vi "Create_Trajectory_Using_TrajectoryLibrary.vi"() -> ()   [LabVIEW 2019]
doc: "This utility creates trajectories based on the robot configuration, constraints and defined waypoints."
uses:
  <vilib>/Rock Robotics/WPI/ThirdParty/JAS_Junk/TrajLib/Trajectory_Library.lvlib
  <vilib>/Utility/xml.llb/Write to XML File(string).vi
  <vilib>/Rock Robotics/WPI/ThirdParty/JAS_Junk/TrajLib/TRANSLATION2D.ctl
  <vilib>/Rock Robotics/WPI/ThirdParty/JAS_Junk/TrajLib/ROTATION2D.ctl
  <vilib>/Rock Robotics/WPI/ThirdParty/JAS_Junk/TrajLib/POSE2D.ctl
  <vilib>/Rock Robotics/WPI/ThirdParty/JAS_Junk/TrajLib/TRAJ_STATE.ctl
  <vilib>/Rock Robotics/WPI/ThirdParty/JAS_Junk/TrajLib/TRAJECTORY.ctl
  <vilib>/Utility/xml.llb/Read From XML File(string).vi
  <vilib>/Rock Robotics/WPI/ThirdParty/JAS_Junk/TrajLib/UTIL_WEIGHTED_WAYPOINT.ctl
  <vilib>/Rock Robotics/WPI/ThirdParty/JAS_Junk/TrajLib/DIFF_DRIVE_KINEMATICS.ctl
  <vilib>/Rock Robotics/WPI/ThirdParty/JAS_Junk/TrajLib/TRAJ_CONSTRAINT_DIIF_DRIVE_KINEMATICS.ctl
  <vilib>/Rock Robotics/WPI/ThirdParty/JAS_Junk/TrajLib/TRAJ_CONSTRAINT_CENTRIPETAL_ACCEL.ctl
  <vilib>/Analysis/Matrix/Datatypes/RealMatrix.ctl
  <vilib>/Analysis/Matrix/NI_Matrix.lvlib
  <vilib>/Rock Robotics/WPI/ThirdParty/JAS_Junk/TrajLib/SWERVE_DRIVE_KINEMATICS.ctl
  <vilib>/Rock Robotics/WPI/ThirdParty/JAS_Junk/TrajLib/TRAJ_CONSTRAINT_SWERVE_DRIVE_KINEMATICS.ctl
  <vilib>/Rock Robotics/WPI/ThirdParty/JAS_Junk/TrajLib/SIMPLE_MOTOR_FF.ctl
  <vilib>/Rock Robotics/WPI/ThirdParty/JAS_Junk/TrajLib/TRAJ_CONSTRAINT_DIIF_DRIVE_VOLTAGE.ctl
  <vilib>/Rock Robotics/WPI/ThirdParty/JAS_Junk/TrajLib/MECA_DRIVE_KINEMATICS.ctl
  <vilib>/Rock Robotics/WPI/ThirdParty/JAS_Junk/TrajLib/TRAJ_CONSTRAINT_MECA_DRIVE_KINEMATICS.ctl
  <vilib>/Rock Robotics/WPI/ThirdParty/JAS_Junk/TrajLib/TRAJ_CONFIG.ctl
  TrajCreateUnitsENUM.ctl
  TrajCreateConfig.ctl
panel:
  in  "End Program":bool
  in  "Tab Control":T1(tab)
  out "Config File Read\nWithout Error":bool
  out "Config File  Read Error":errorcluster
  out "Read Config File Comment":string
  in  "Read Config File Name":path
  in  "ReadConfigFile":bool
  in  "Field Selector":string(combo)
  in  "Units Selector":T2
  in  "MaxVelocity":dbl=50.0 format="%17.1f"
  in  "MaxAcceleration":dbl=40.0 format="%17.1f"
  out "MaxVelocity M/S":dbl=2.0 format="%17.4f"
  out "MaxAcceleration M/S^2":dbl=1.3 format="%17.4f"
  in  "Right Rear":T3={"X"=-0.5, "Y"=0.5} {"Y" format="%14.3f"; "X" format="%14.3f"}
  in  "Left Rear":T3={"X"=-0.5, "Y"=-0.5} {"Y" format="%14.3f"; "X" format="%14.3f"}
  in  "Right Front":T3={"X"=0.5, "Y"=0.5} {"Y" format="%14.3f"; "X" format="%14.3f"}
  in  "Left Front":T3={"X"=0.5, "Y"=-0.5} {"Y" format="%14.3f"; "X" format="%14.3f"}
  in  "Use Centripetal\nAcceleration\nConstaint":bool=TRUE
  out "Max Cent Accel M/S^2":dbl=1.0 format="%20.4f"
  in  "Max Cent Accel":dbl=20.0 format="%20.1f"
  in  "Use Diff Drive\nKinematic\nConstraint":bool=TRUE
  out "Wheelbase Width M":dbl=0.66 format="%20.4f"
  in  "Wheelbase Width":dbl=20.866 format="%20.1f"
  in  "Max Voltage":dbl=12.0 format="%20.4f"
  in  "SIMPLE_MOTOR_FF":T4={"Ks"=0.9, "Kv"=8.74, "Ka"=1.92} {"Ka" format="%13.4f"; "Kv" format="%13.4f"; "Ks" format="%13.4f"}
  in  "Use Diff Drive\nVoltage\nConstraint":bool=TRUE
  in  "Wheels":T3[](array[typedef])=[{"X"=0.5, "Y"=-0.5}, {"X"=0.5, "Y"=0.5}, {"X"=-0.5, "Y"=0.5}, {"X"=-0.5, "Y"=-0.5}] {"Y" format="%14.3f"; "X" format="%14.3f"}
  in  "Use Swerve Drive\nKinematics\nConstraint":bool
  in  "Use Mecanum \nDrive Kinematics\nConstraint":bool
  out "Left Front M":T3 {"Y" format="%14.3f"; "X" format="%14.3f"}
  out "Right Front M":T3 {"Y" format="%14.3f"; "X" format="%14.3f"}
  out "Left Rear M":T3 {"Y" format="%14.3f"; "X" format="%14.3f"}
  out "Right Rear M":T3 {"Y" format="%14.3f"; "X" format="%14.3f"}
  out "SIMPLE_MOTOR_FF M":T4 {"Ka" format="%13.4f"; "Kv" format="%13.4f"; "Ks" format="%13.4f"}
  out "Wheels M":T3[](array[typedef]) {"Y" format="%14.3f"; "X" format="%14.3f"}
  in  "WayPoints":T5[](array[typedef])=[{"X"=15.0, "Y"=105.0, "ANGLE"=-45.0, "WEIGHT"=12.0}, {"X"=105.0, "Y"=65.0, "ANGLE"=0.0, "WEIGHT"=12.0}, {"X"=210.0, "Y"=106.0, "ANGLE"=45.0, "WEIGHT"=12.0}, {"X"=350.0, "Y"=105.0, "ANGLE"=-45.0, "WEIGHT"=12.0}] {"WEIGHT" format="%13.3f"; "ANGLE" format="%13.3f"; "Y" format="%13.3f"; "X" format="%13.3f"}
  in  "Spline Type":enum32{"Radio Selection 1", "Radio Selection 2"}(radio)
  in  "Reverse":bool
  in  "UseWeights":bool
  in  "Calculate\nTrajectory":bool
  out "Trajectory\nCompleted\nError Free":bool
  out "Trajectory calculation error":errorcluster
  out "Position":cluster{dbl[], dbl[]}[](graph)
  out "Field Display":T6(plugin-control)
  out "Trajectory Data":cluster{dbl[], dbl[]}[](graph)
  out "differential \ndrive \nmax speed":dbl format="%15.1f"
  out "Traj States\nSize":i32
  out "Trajectory States":T7[](array[typedef]) {"POSE"."ROTATION"."SIN" format="%13.4f"; "POSE"."ROTATION"."COS" format="%13.4f"; "POSE"."ROTATION"."VALUE" format="%13.4f"; "POSE"."TRANSLATION"."Y" format="%14.3f"; "POSE"."TRANSLATION"."X" format="%14.3f"}
  in  "Trajectory JSON File Name":path
  out "JSON File Saved\nWithout Error":bool
  out "Write CSV File Error":errorcluster
  in  "PathWeaver Length Units":T10(radio)
  in  "WriteJSONFile":bool
  out "CSV File Saved\nWithout Error":bool
  in  "Trajectory Type":enum32{"Radio Selection 1", "Radio Selection 2"}(radio)
  out "Write Trajectory\nFile Error":errorcluster
  in  "Trajectory File Comment":string
  in  "Trajectory CSV File Name":path
  in  "WriteTrajFile":bool
  out "Config File Saved\nWithout Error":bool
  out "Write Config FIle Error":errorcluster
  in  "Write Config File Comment":string
  in  "Write Config File Name":path
  in  "WriteConfigFile":bool
  # "Create Trajectory  (Use LabVIEW trajectory library)"
  # "Instructions:  \n----------------\n\nThis utility will create a trajectory, show the data on the various tabs, and optionally write a \"field absolute\" or \"robot relative\" trajectory to a file. \nTo use this utility:\n\n1) Read all of these instructions!\n2) Define the robot's physical data on the \"Robot Data\" tab.  \n3) Define the robot's movement constraints on the \"Constraints\" page.  \n4) Define the trajectory on the \"Define/Create Trajectory\" tab.  These are the beginning and ending positions/headings, and internal positions/headings.  \n    Cubic splines only use the first and last \"angle\".  The other internal \"angles\" are calculated.  Quintic splines use all the defined angles.\n5) Press the \"Calculate Trajectory\".  If a good trajectory was calculated it will be displayed.  If no errors are generated the Trajectory Complete\n    light will be on.  Errors will be displayed in the error indicator.  The path can be recalculated many times before performing any other action.\n\nAfter a Trajectory has been calculated, the \"trajectory can be written to a file.  The absolute path is converted to a robot relative trajectory.  To do this:\n1) Enter a comment to be included in the file.  Anything can be entered.\n2) Select the file name.\n3) Press \"Create Trajectory File\"  If an error occurs it will be displayed in the File Creation Error indicator.\n\nNotes:\n--------\n- All the robot parameters, path, and field dimensions are in UNITS, and DEGREES.  Select UNITS from the \"Robot Data\" page.  The resulting  \n  trajectory is converted to METERS, and RADIANS to match the rest of this library!\n- The trajectory library is the same as the WPILIB spline and trajectory library for Java and C++.\n- 2019 playing field size - width: 26 ft 11.25 In = 323.25 in , length: 52 ft 5.25 in = 629.25 in  (I didn't verify this for the 2020 version.)"
  # "Read Trajectory Waypoints and Configuration from File"
  # "ROBOT DATA"
  # "UNITS/SEC"
  # "Meters/SEC"
  # "UNITS/SEC^2"
  # "Meters/SEC^2"
  # "Simulated robot max speed is: 68.266 Inches/Second"
  # "UTILITY CONFIGURATION"
  # "Diff Kinematics Constraint"
  # "Centripetal Accel Constraint"
  # "Diff Voltage Constraint"
  # "UNITS"
  # "UNITS/SEC^2"
  # "VOLTS"
  # "METERS"
  # "METERS/SEC^2"
  # "Distance is:\nUNITS"
  # "Simulated robot wheelbase is 20.87 in"
  # "Ks = Volts\nKv = VoltSec/Meter\nKa = Volt(Sec^2)/Meter"
  # "Swerve Kinematics Constraint"
  # "Mechanum Kinematics Constraint"
  # "Values\nare \nUNITS"
  # "Values\nare \nUNITS"
  # "TRAJECTORY DEFINITION"
  # "To delete array elements or the entire array, right click on the array or element, select Data Operations, then select the action to be performed."
  # "UNITS, UNITS, DEGREES, SCALAR"
  # "INCHES/SEC"
  # "Write Trajectory to File   -   CSV, and / or JSON"
  # "Write Trajectory Waypoints and Configuration to File"
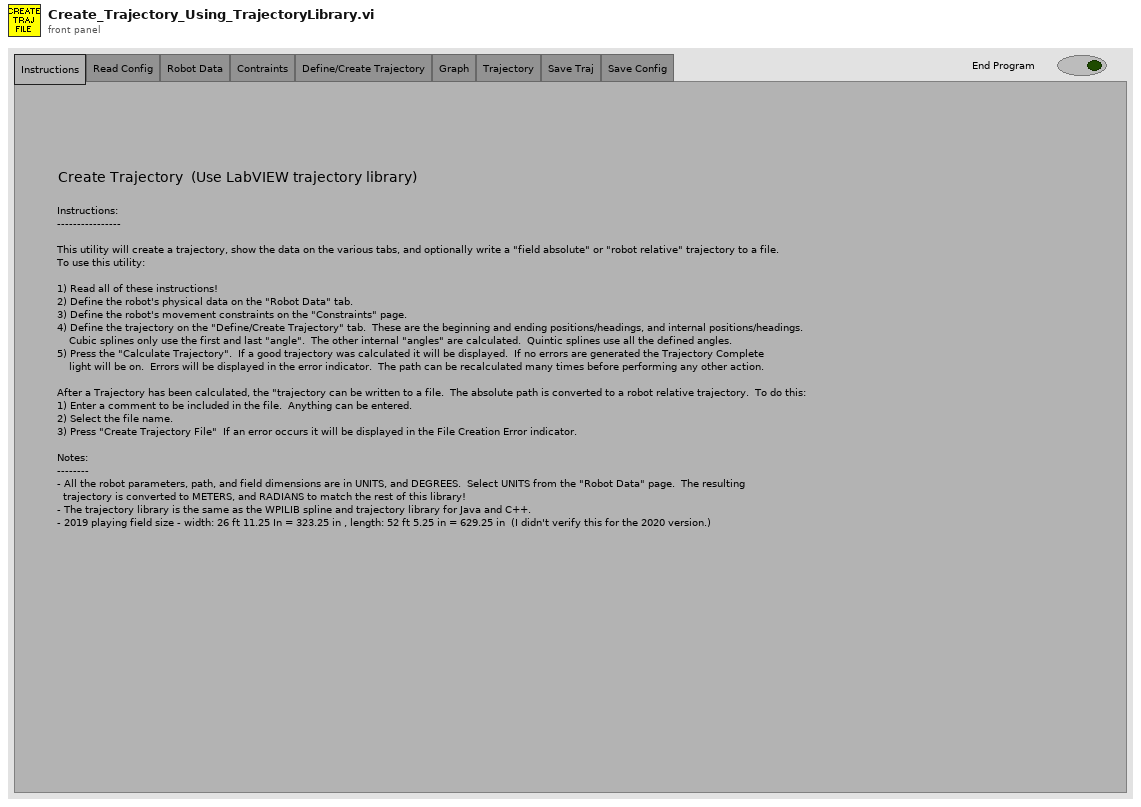
[diagram p1: front panel]
types:
  T1 = enum32{"Instructions", "Read Config", "Robot Data", "Contraints", "Define/Create Trajectory", "Graph", "Trajectory", "Save Traj", "Save Config"}
  T2 = typedef "TrajCreateUnitsENUM.ctl" = enum16{"Inches", "Feet", "Centimeters", "Meters"}
  T3 = typedef "Trajectory_Library.lvlib/TRANSLATION2D.ctl" = cluster{"X":dbl, "Y":dbl}
  T4 = typedef "Trajectory_Library.lvlib/SIMPLE_MOTOR_FF.ctl" = cluster{"Ks":dbl, "Kv":dbl, "Ka":dbl}
  T5 = typedef "Trajectory_Library.lvlib/UTIL_WEIGHTED_WAYPOINT.ctl" = cluster{"X":dbl, "Y":dbl, "ANGLE":dbl, "WEIGHT":dbl}
  T6 = typedef "IMAQ Image.ctl" = refnum<image>
  T7 = typedef "Trajectory_Library.lvlib/TRAJ_STATE.ctl" = cluster{"TimeSeconds":dbl, "Velocity":dbl, "Acceleration":dbl, "POSE":T8, "Curvature":dbl}
  T8 = typedef "Trajectory_Library.lvlib/POSE2D.ctl" = cluster{"TRANSLATION":T3, "ROTATION":T9}
  T9 = typedef "Trajectory_Library.lvlib/ROTATION2D.ctl" = cluster{"VALUE":dbl, "COS":dbl, "SIN":dbl}
  T10 = enum32{"Radio Selection 1", "Radio Selection 2", "Radio Selection 3", "Radio Selection 4", "Radio Selection 5"}
  T11 = typedef "Image Type" = u32
  T12 = enum8{"Enabled", "Disabled", "Disabled and Grayed Out"}
  T13 = typedef "Trajectory_Library.lvlib/TRAJECTORY.ctl" = cluster{"TotalTImeSecs":dbl, "States":T7[]}
  T14 = typedef "TrajCreateConfig.ctl" = cluster{"Write Config File Name":path, "Write Config File Comment":string, "WayPoints":T5[], "TRAJECTORY_CONFIG":T15, "IsCubic":bool, "Units Selector":T2, "UseWeights":bool}
  T15 = typedef "Trajectory_Library.lvlib/TRAJ_CONFIG.ctl" = cluster{"MaxVelocity":dbl, "Max Acceleration":dbl, "StartVelocity":dbl, "End Velocity":dbl, "Reversed":bool, "DiffDrKineConstntDefined":bool, "CentAcellConstntDefined":bool, "DiffDrVoltConstntDefined":bool, "DIFF_DRIVE_KINE_CONSTRAINT":T16, "CENTRIPETAL_ACCEL_CONSTRAINT":T18, "SwerveDrKineConstntDefined":bool, "SWERVE_DRIVE_KINE_CONSTRAINT":T19, "DIFF_DRIVE_VOLTAGE_CONSTRAINT":T22, "MECANUM_DRIVE_KINE_CONSTRAINT":T23, "MecanumDrKineConstntDefined":bool}
  T16 = typedef "Trajectory_Library.lvlib/TRAJ_CONSTRAINT_DIIF_DRIVE_KINEMATICS.ctl" = cluster{"Max Speed (M/S)":dbl, "DIFF_DRIVE_KINEMATICS":T17}
  T17 = typedef "Trajectory_Library.lvlib/DIFF_DRIVE_KINEMATICS.ctl" = cluster{"TrackWidth_Meters":dbl}
  T18 = typedef "Trajectory_Library.lvlib/TRAJ_CONSTRAINT_CENTRIPETAL_ACCEL.ctl" = cluster{"Max Cent Accel":dbl}
  T19 = typedef "Trajectory_Library.lvlib/TRAJ_CONSTRAINT_SWERVE_DRIVE_KINEMATICS.ctl" = cluster{"Max Speed (M/S)":dbl, "SwerveKinematics":T20}
  T20 = typedef "Trajectory_Library.lvlib/SWERVE_DRIVE_KINEMATICS.ctl" = cluster{"NumModules":i32, "InverseKinematics":T21, "ForwardKinematics":T21, "Modules":T3[], "PrevCoR":T3}
  T21 = typedef "NI_Matrix.lvlib/RealMatrix.ctl" = dbl[][]
  T22 = typedef "Trajectory_Library.lvlib/TRAJ_CONSTRAINT_DIIF_DRIVE_VOLTAGE.ctl" = cluster{"Max Voltage":dbl, "DIFF_DRIVE_KINEMATICS":T17, "SIMPLE_MOTOR_FF":T4}
  T23 = typedef "Trajectory_Library.lvlib/TRAJ_CONSTRAINT_MECA_DRIVE_KINEMATICS.ctl" = cluster{"Max Speed (M/S)":dbl, "MECA_DRIVE_KINEMATICS":T24}
  T24 = typedef "Trajectory_Library.lvlib/MECA_DRIVE_KINEMATICS.ctl" = cluster{"FrontLeft":T3, "FrontRight":T3, "RearLeft":T3, "RearRight":T3, "InverseKinematics":T21, "ForwardKinematics":T21, "PrevCoR":T3}
  T25 = typedef "TrajectoryUtils_Field_Info.ctl" = cluster{"FIeld_File_Name":string, "Top_Left_X":i32, "Top_Left_Y":i32, "Bottom_Right_X":i32, "Bottom_Right_Y":i32, "Field_Size_X":dbl, "Field_Size_Y":dbl, "FIeld_Size_Units":string}
  T26 = typedef "Trajectory_Library.lvlib/WEIGHTED_WAYPOINT.ctl" = cluster{"TRANSLATION":T3, "ROTATION":T9, "SCALAR":dbl}
  T27 = typedef "Trajectory_Library.lvlib/SPLINE_CTRL_VECTOR.ctl" = cluster{"Xs":dbl[], "Ys":dbl[]}
  T28 = typedef "Trajectory_Library.lvlib/CHASSIS_SPEEDS.ctl" = cluster{"vX":dbl, "vY":dbl, "vOmega":dbl}
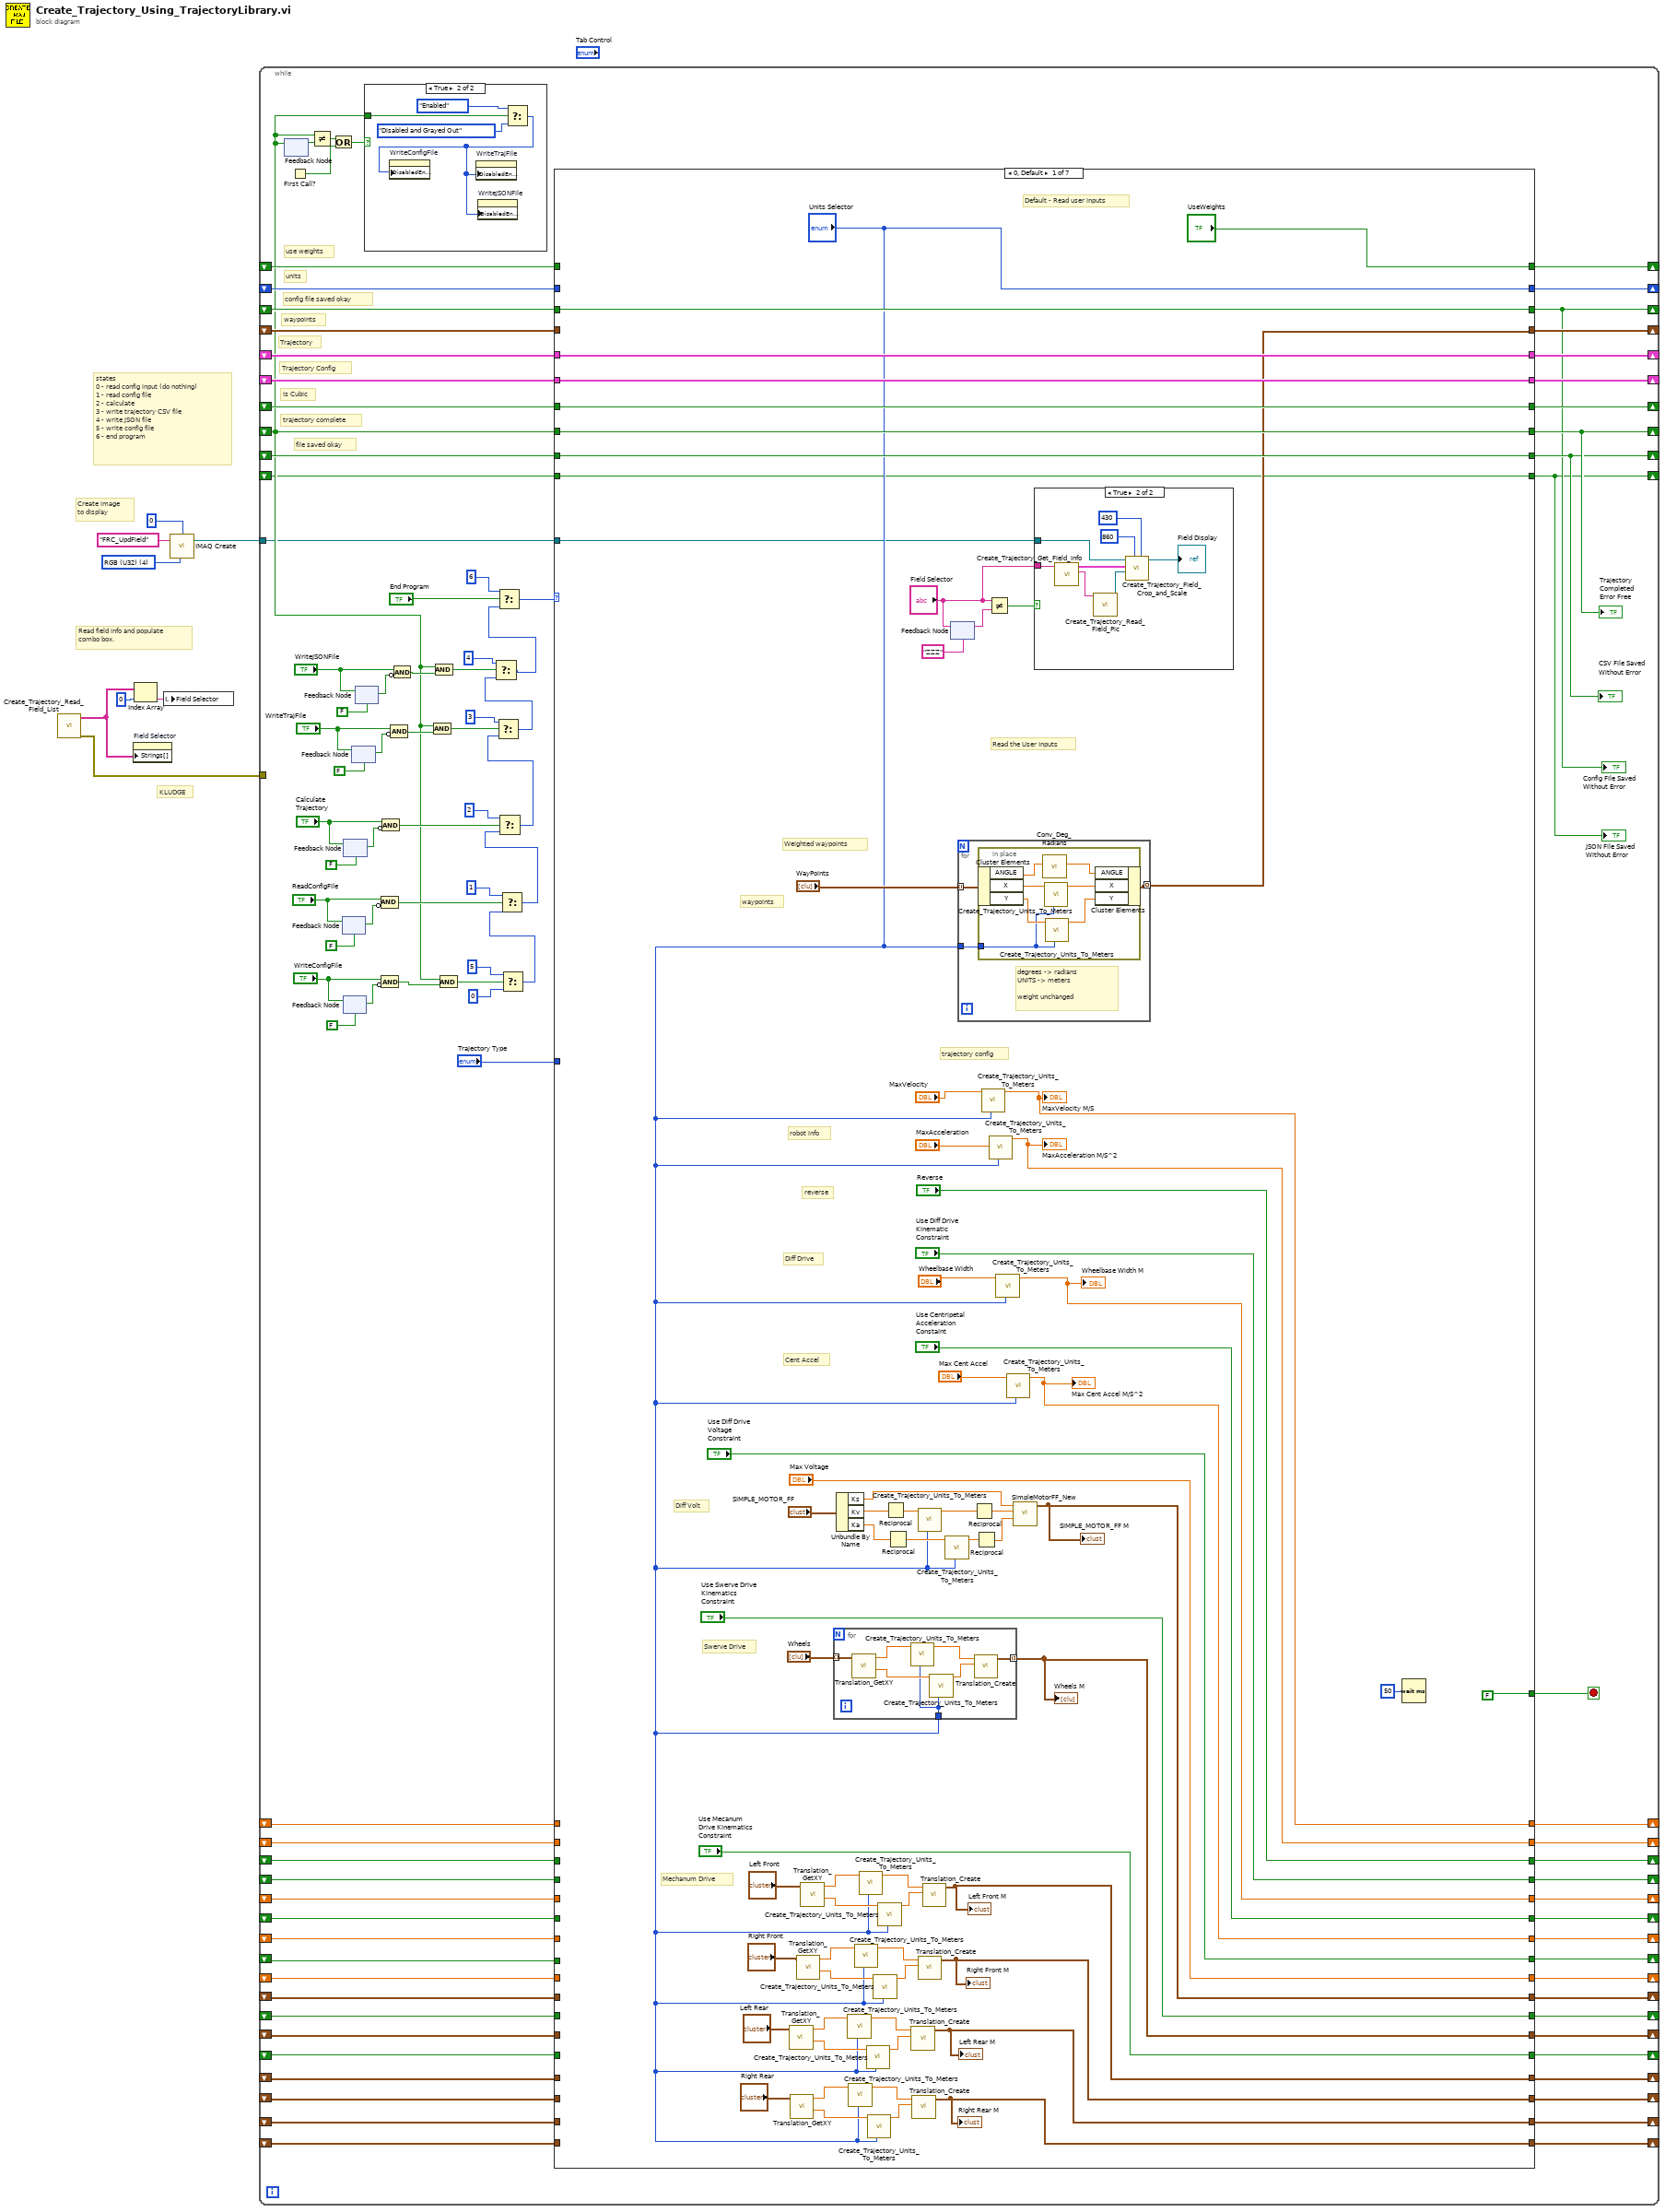
[diagram p0: block diagram]
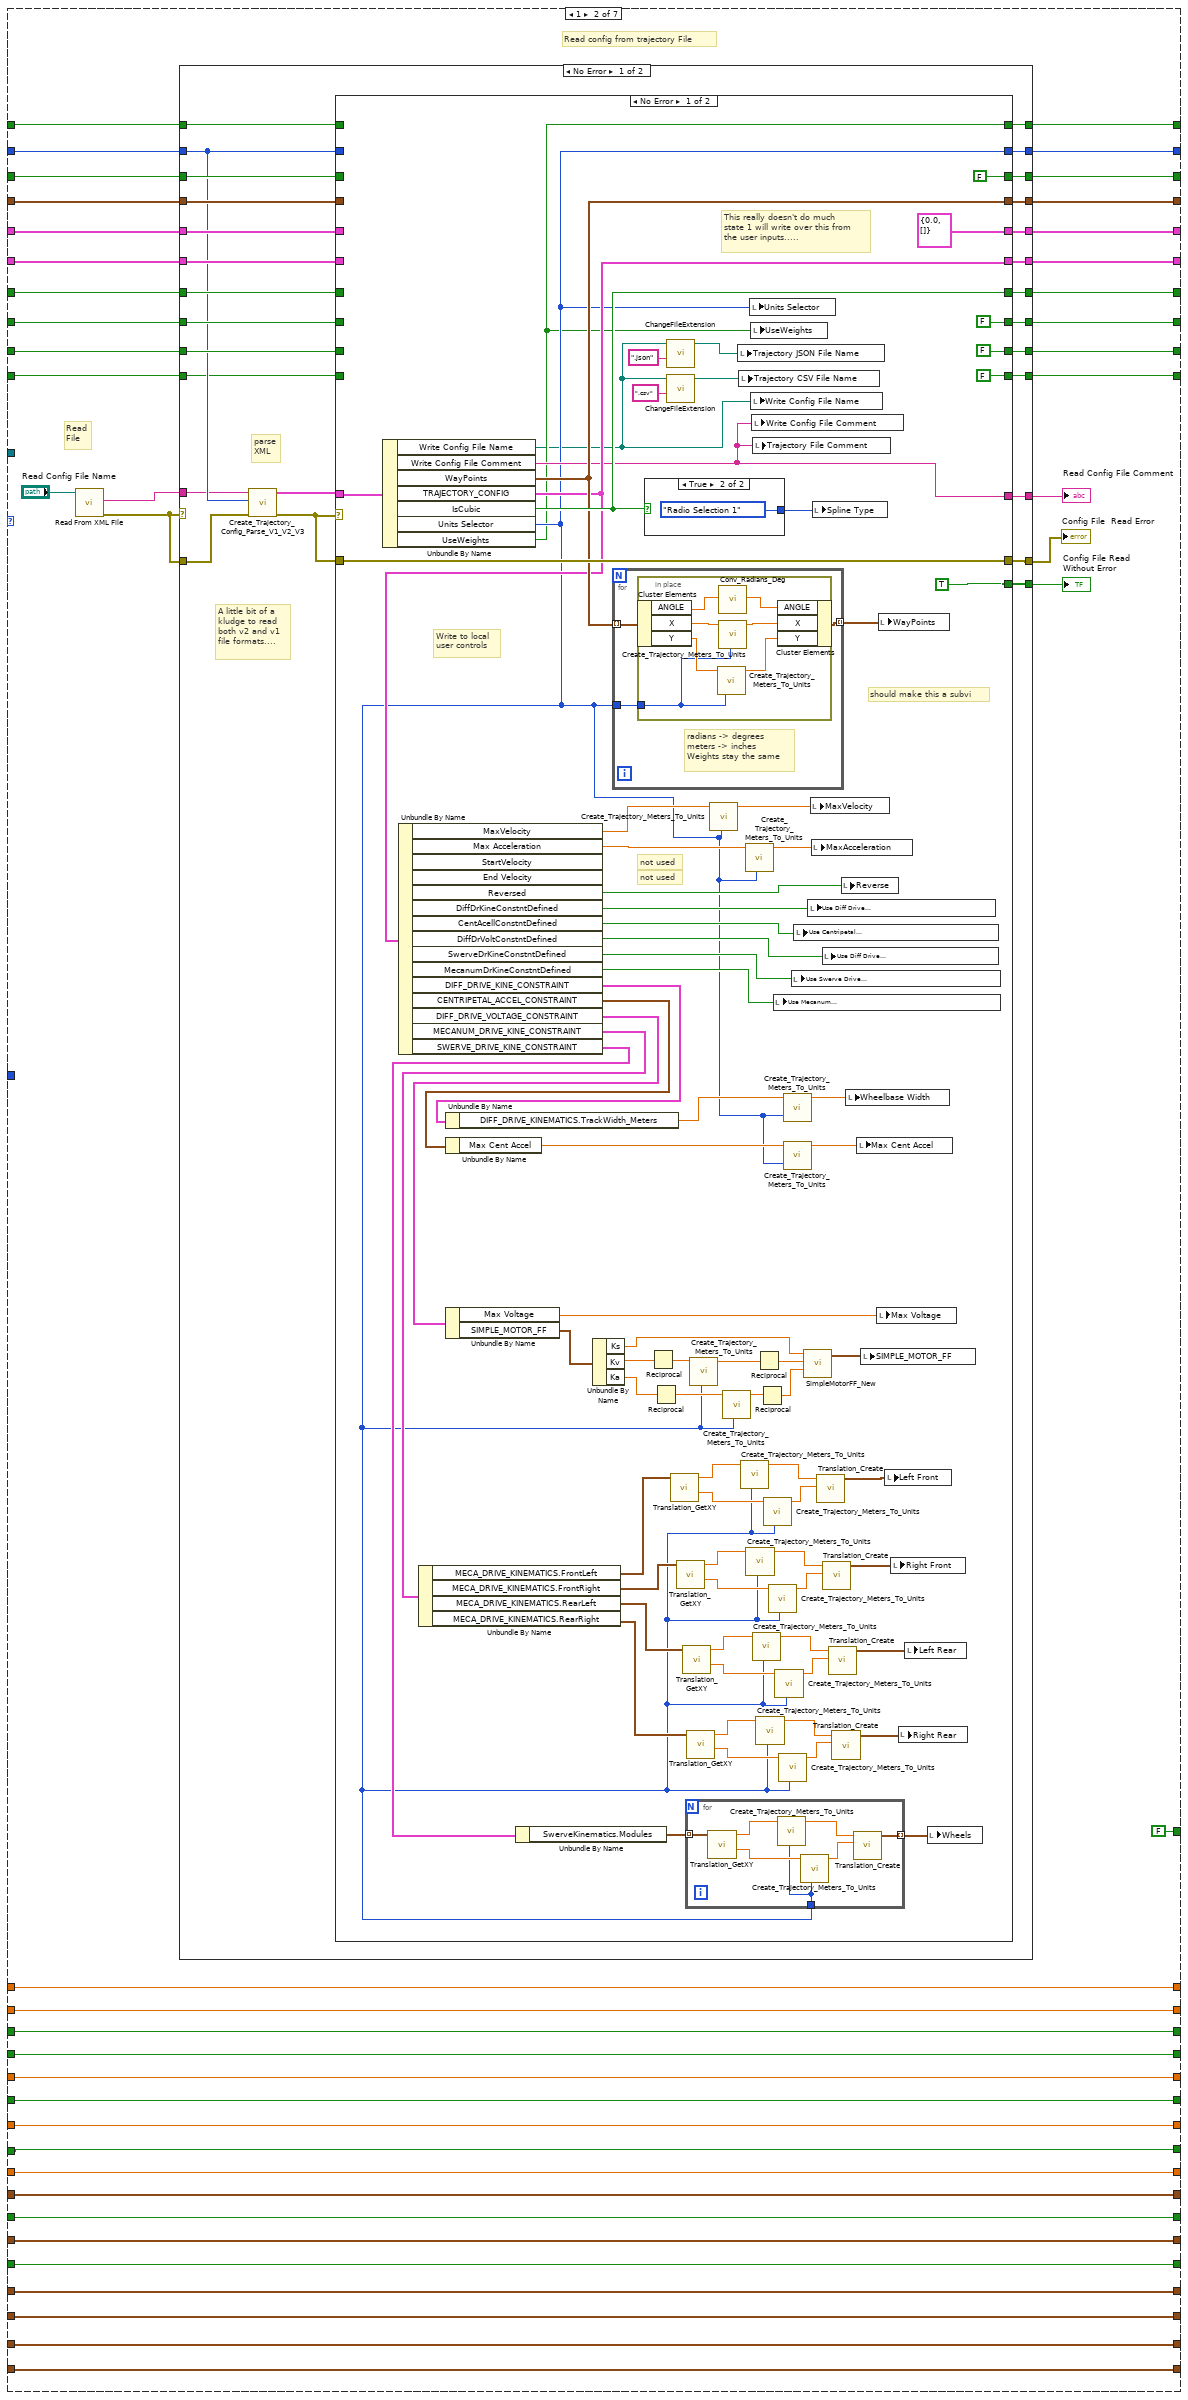
[diagram p4: hidden frame]
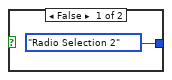
[diagram p5: hidden frame]
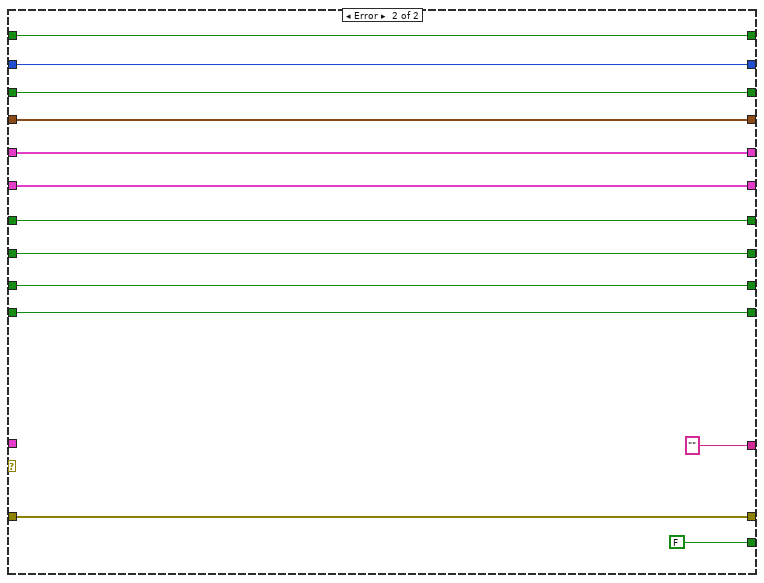
[diagram p6: hidden frame]
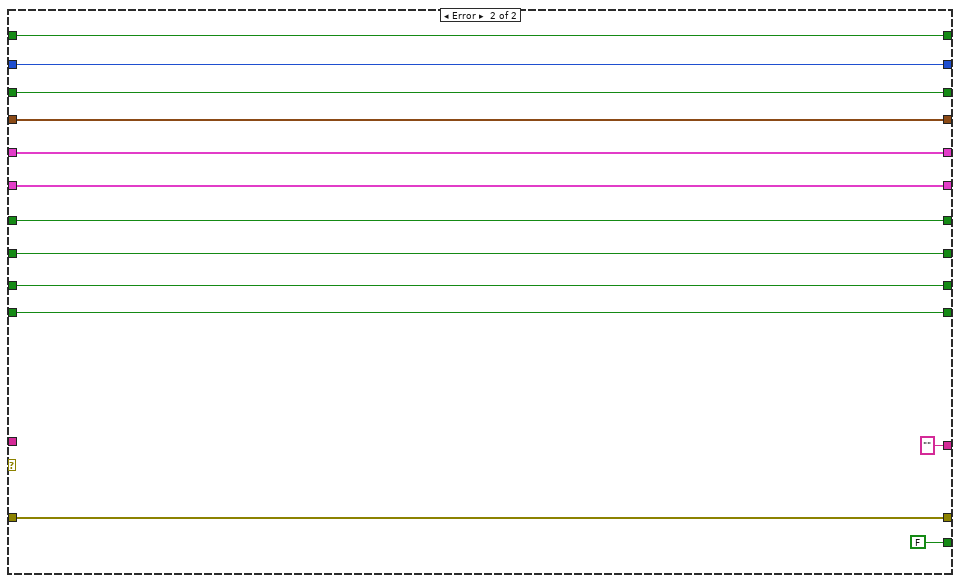
[diagram p7: hidden frame]
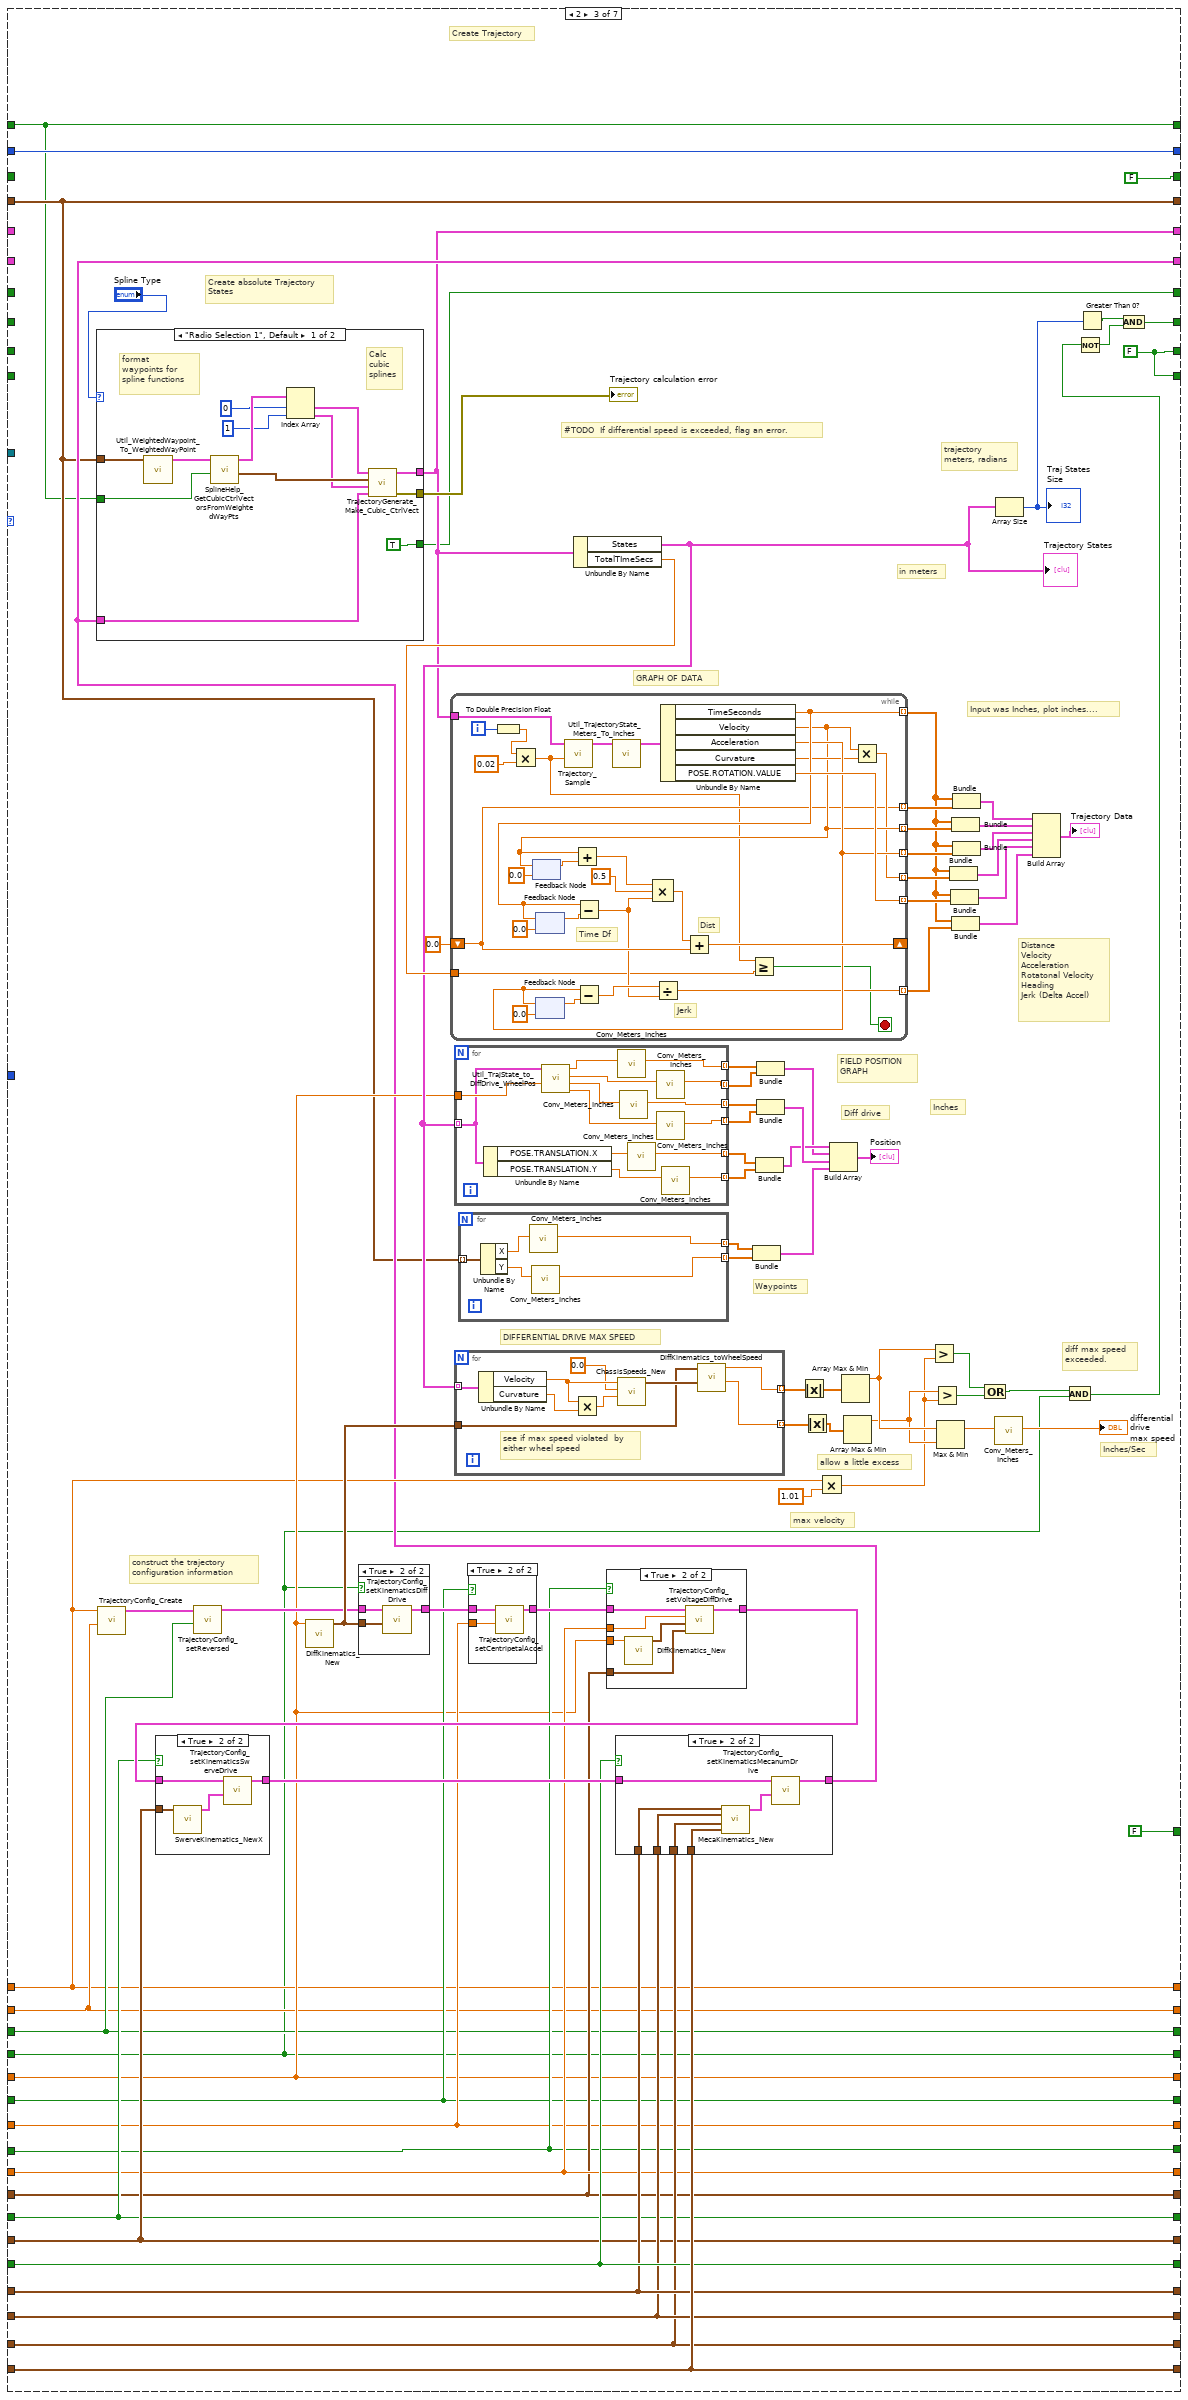
[diagram p8: hidden frame]
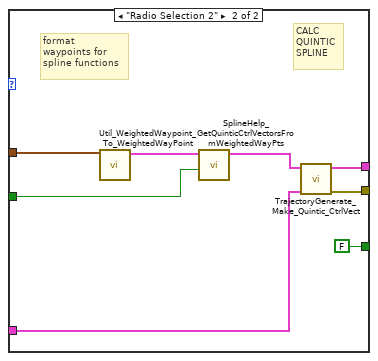
[diagram p12: hidden frame]
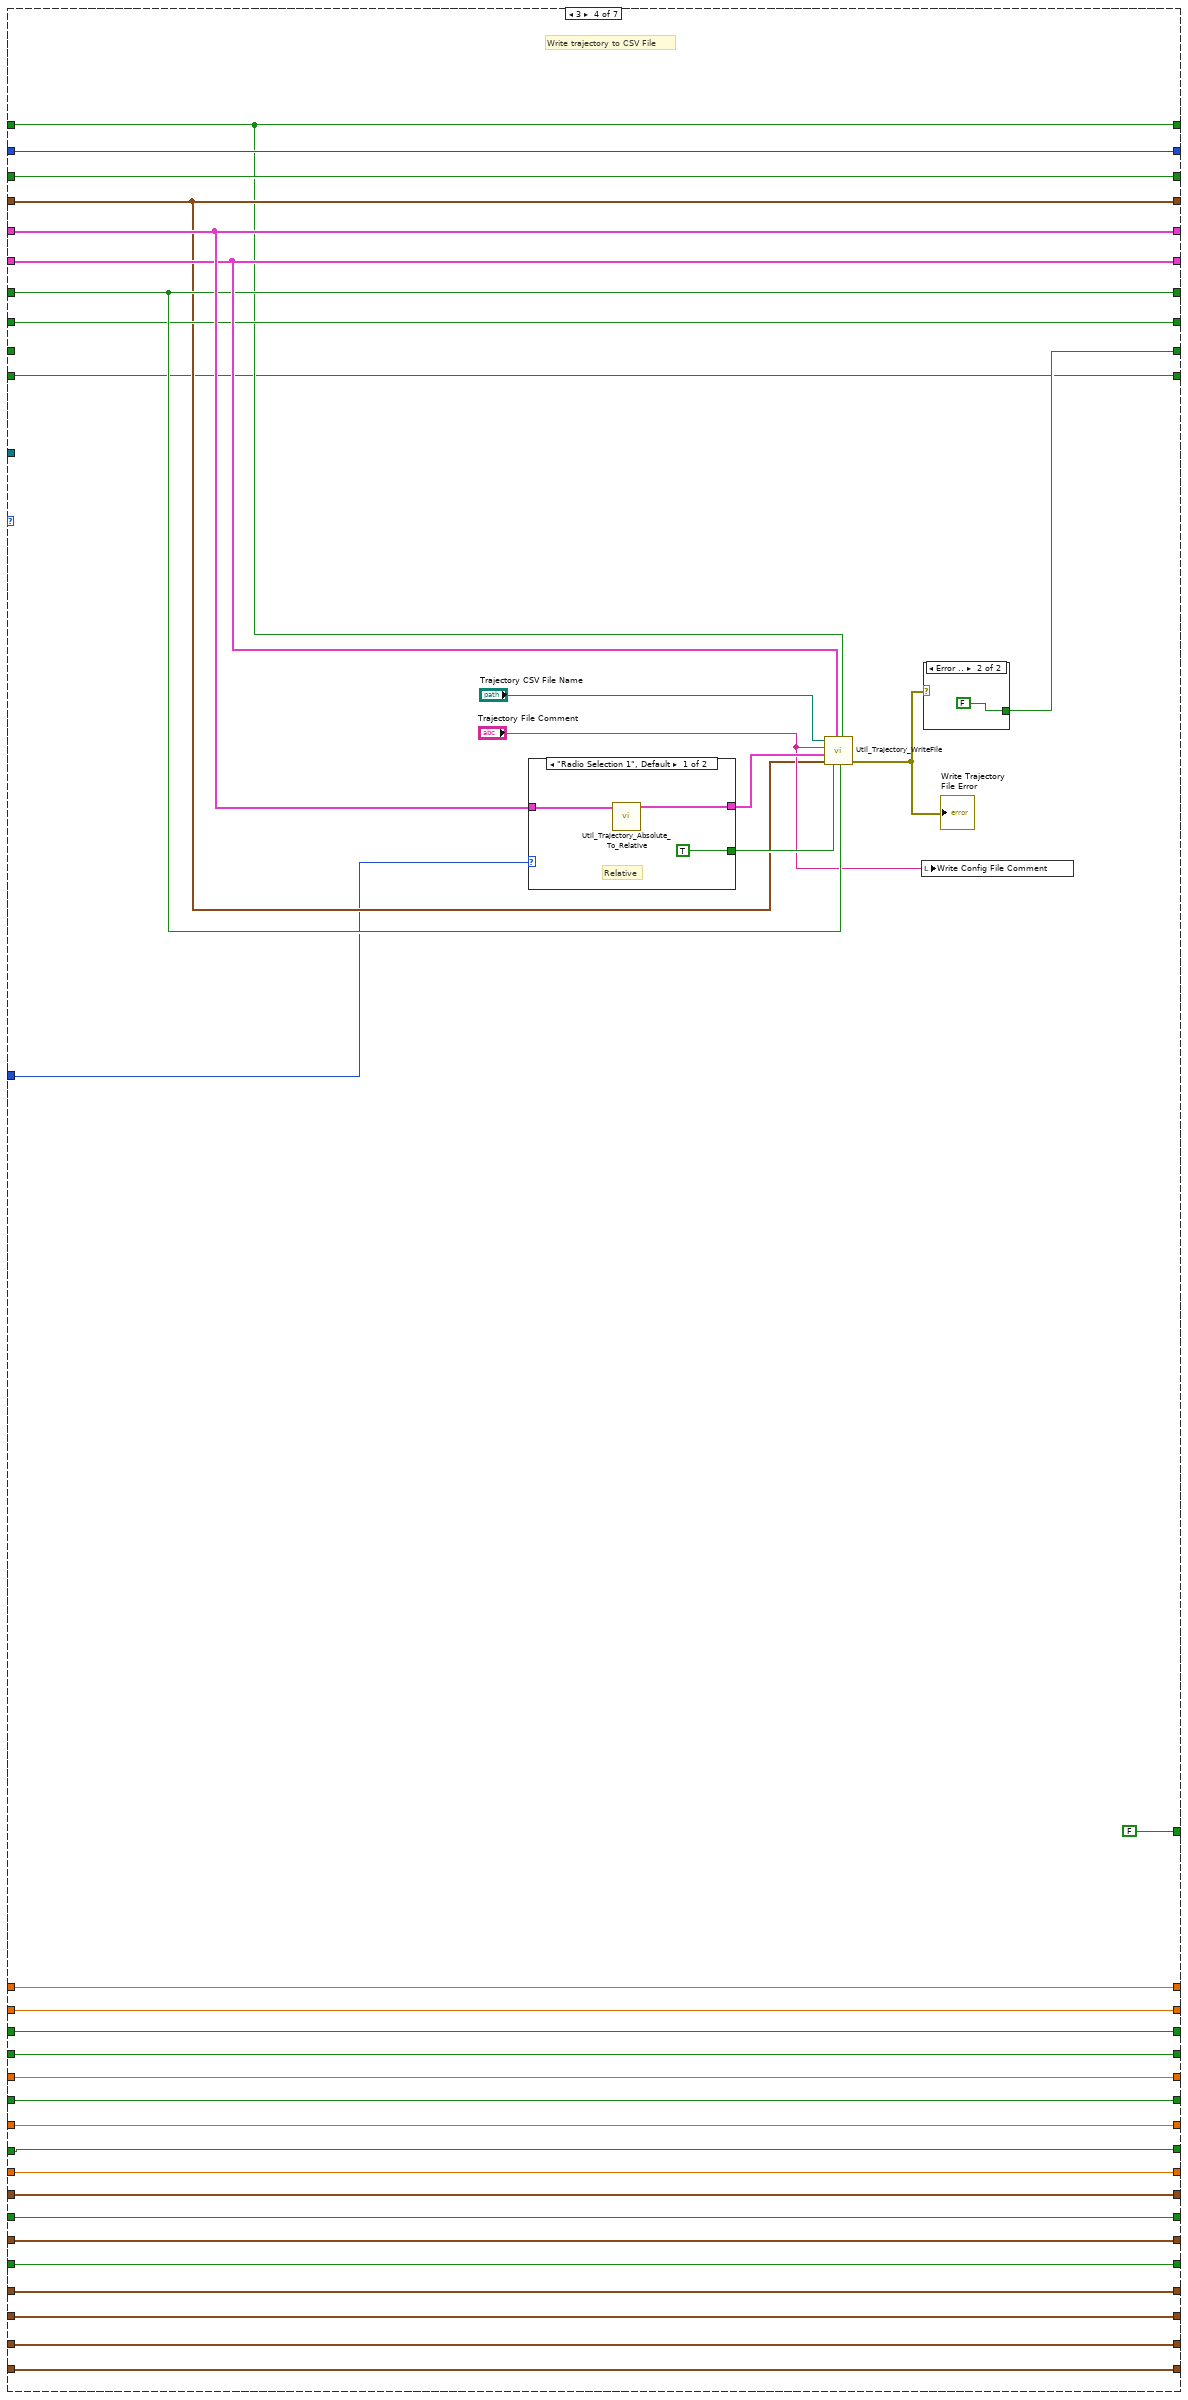
[diagram p15: hidden frame]
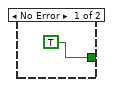
[diagram p16: hidden frame]
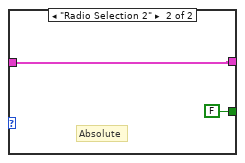
[diagram p17: hidden frame]
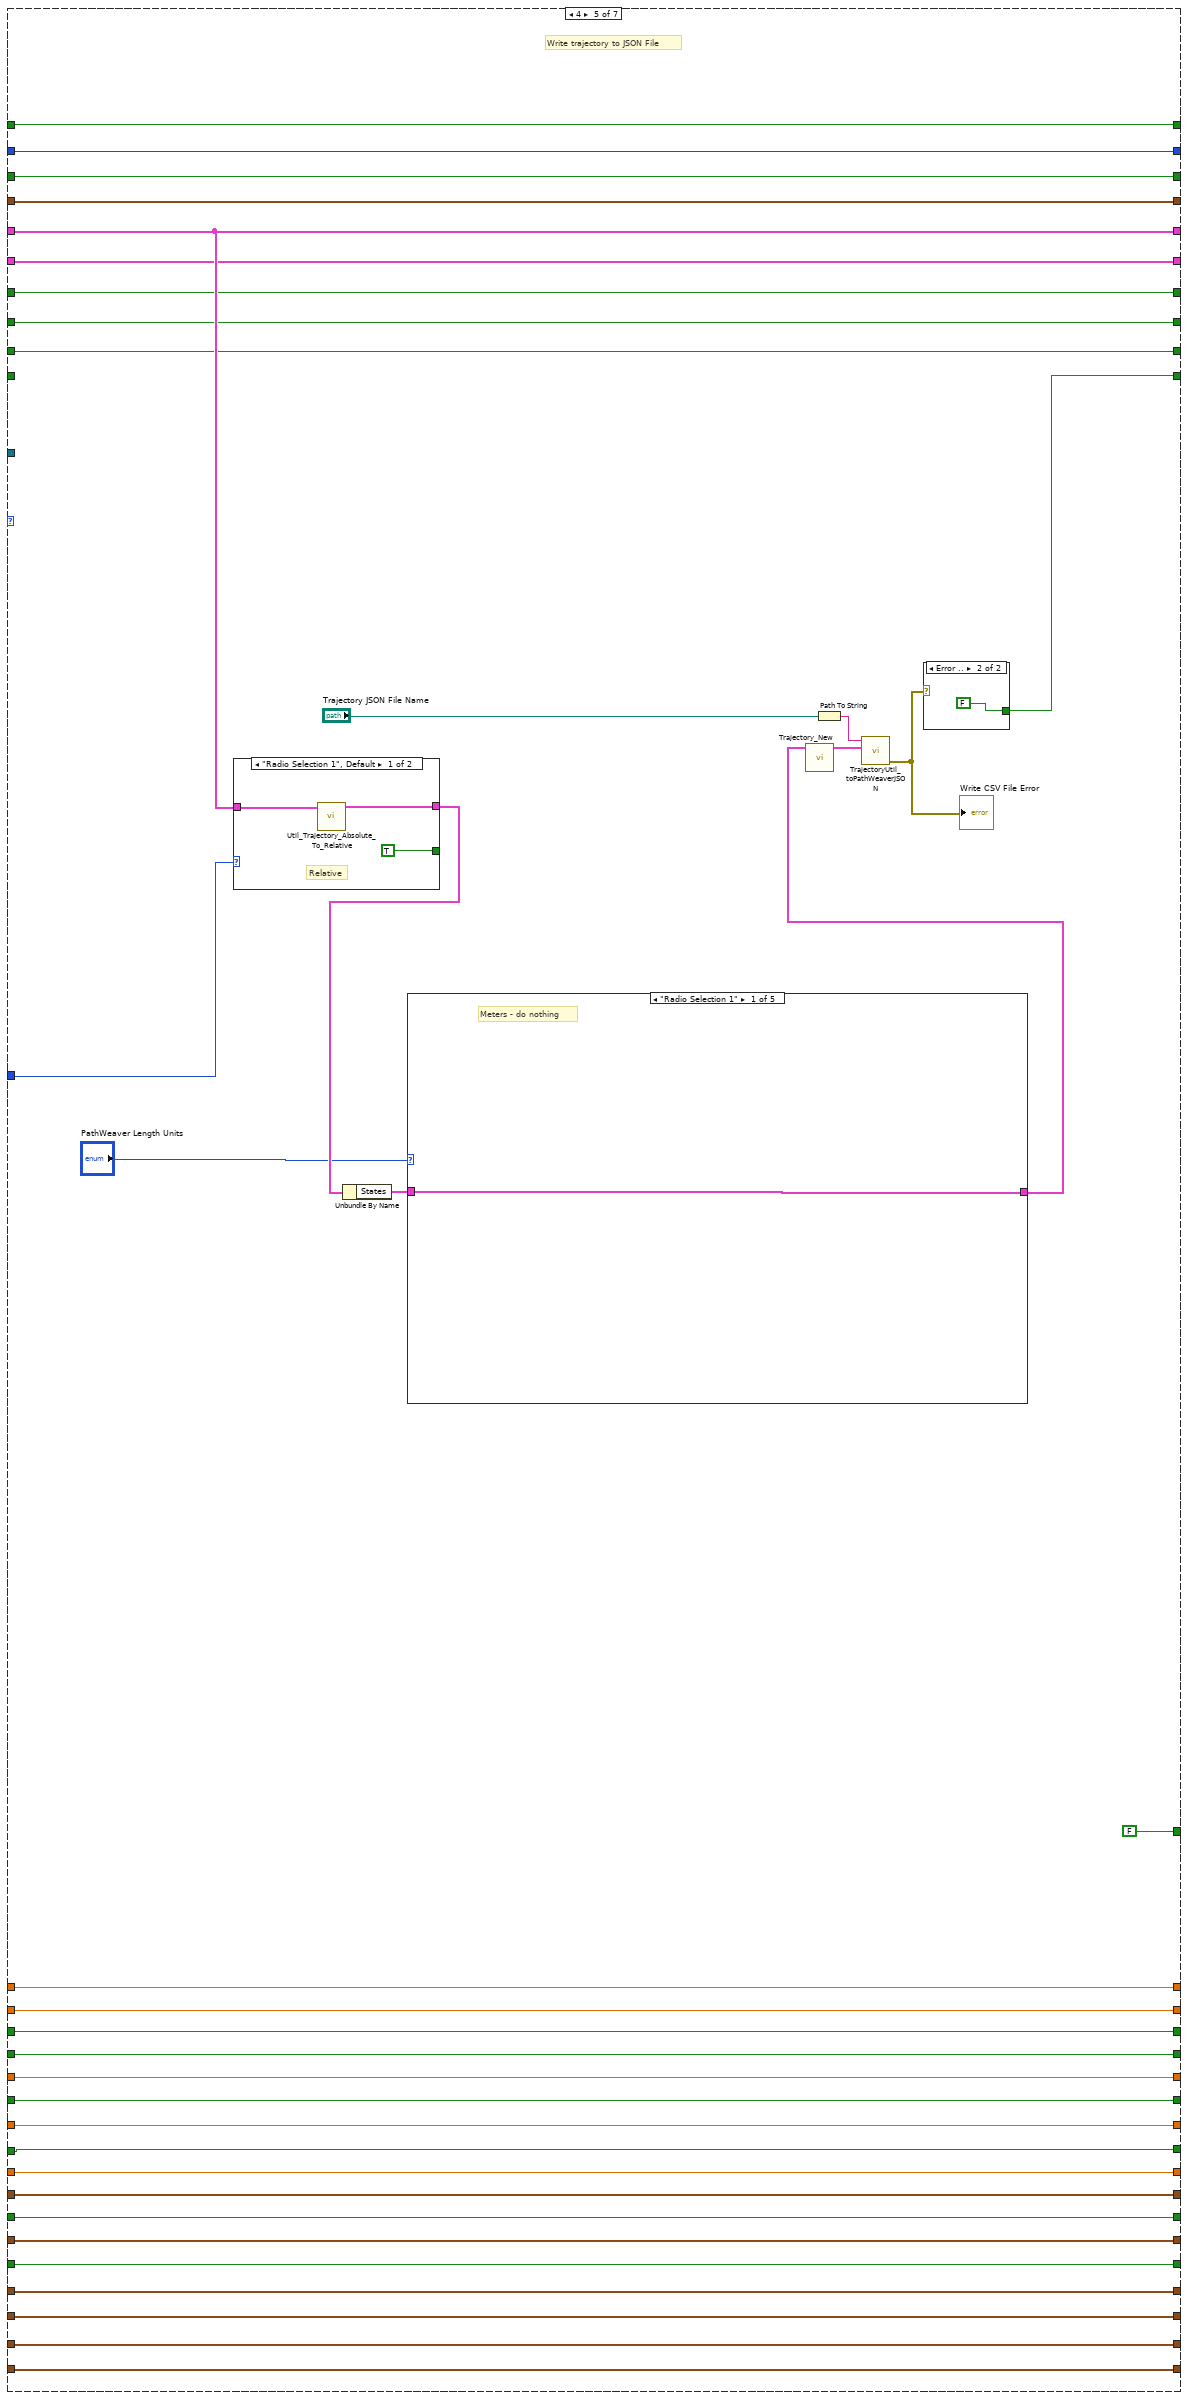
[diagram p18: hidden frame]
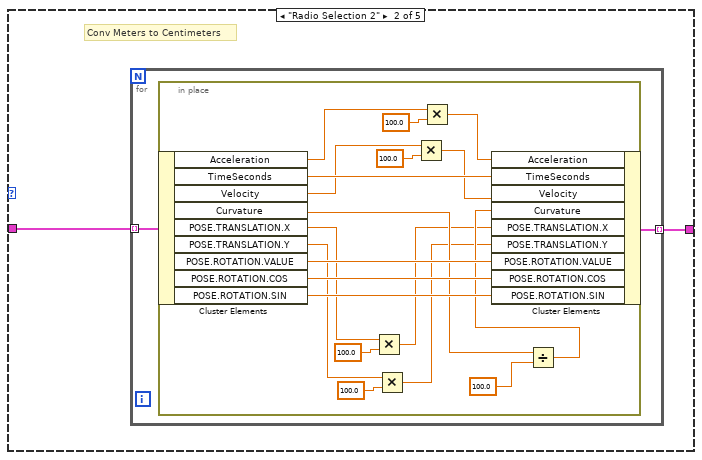
[diagram p19: hidden frame]
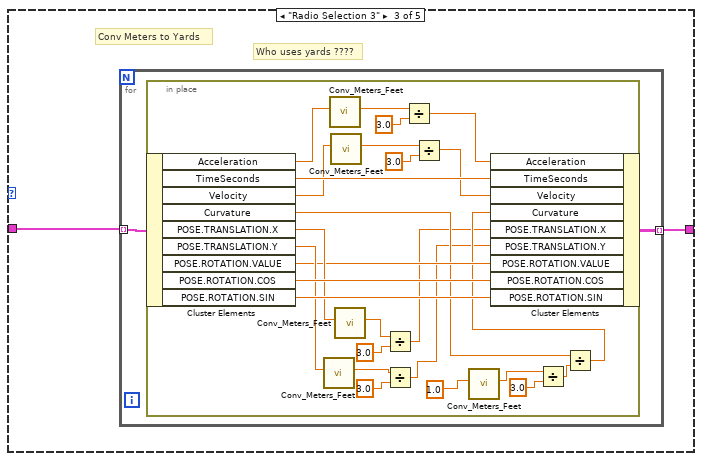
[diagram p20: hidden frame]
diagram:
  w2 = T11 4 items=["Grayscale (U8)", "Grayscale (I16)", "Grayscale (SGL)", "Complex (CSG)", "RGB (U32)", "HSL (U32)", "RGB (U64)", "Grayscale (U16)"] ("Image Type")
  # "Create image \nto display"
  # "KLUDGE"
  # "Read field info and populate\ncombo box."
  # "states\n0 - read config input (do nothing)\n1 - read config file\n2 - calculate\n3 - write trajectory CSV file\n4 - write JSON file\n5 - write config file\n6 - end program"
  n1 = call "Create_Trajectory_Read_Field_List.vi"() -> ("error out"=w5:errorcluster, "section names"=w6:string[])  [unwired: 10 in]
  n2 = property on="Field Selector" class="CmbBox"("Strings[]"=w6) -> ()  [unwired: 2 in, 2 out]
  n3 = Index Array(array=w6, index=0) -> (element=w7:string)
  n4 = local write "Field Selector"(w7) -> ()
  n5 = call "IMAQ Create"("Border Size"=0, "Image Name"="FRC_UpdField", "Image Type"=w2) -> ("New Image"=w1:T6)  [unwired: 2 in, 1 out]
  n6 = while {
    shift-right: [w97] -> _
    shift-left: _ -> [w96]
    shift-right: [w95] -> _
    shift-left: _ -> [w94]
    shift-right: [w79] -> _
    shift-left: _ -> [w80]
    shift-right: [w82] -> _
    shift-left: _ -> [w81]
    shift-right: [w78] -> _
    shift-left: _ -> [w17]
    shift-right: [w74] -> _
    shift-left: _ -> [w75]
    shift-right: [w64] -> _
    shift-left: _ -> [w69]
    shift-right: [w73] -> _
    shift-left: _ -> [w68]
    shift-right: [w65] -> _
    shift-left: _ -> [w72]
    shift-right: [w66] -> _
    shift-left: _ -> [w71]
    shift-right: [w67] -> _
    shift-left: _ -> [w70]
    shift-right: [w63] -> _
    shift-left: _ -> [w61]
    shift-right: [w62] -> _
    shift-left: _ -> [w60]
    shift-right: [w57] -> _
    shift-left: _ -> [w58]
    shift-right: [w56] -> _
    shift-left: _ -> [w59]
    shift-right: [w54] -> _
    shift-left: _ -> [w55]
    shift-right: [w50] -> _
    shift-left: _ -> [w52]
    shift-right: [w51] -> _
    shift-left: _ -> [w53]
    shift-right: [w47] -> _
    shift-left: _ -> [w49]
    shift-right: [w46] -> _
    shift-left: _ -> [w48]
    shift-right: [w40] -> _
    shift-left: _ -> [w43]
    shift-right: [w41] -> _
    shift-left: _ -> [w44]
    shift-right: [w42] -> _
    shift-left: _ -> [w45]
    shift-right: [w27] -> _
    shift-left: _ -> [w26]
    shift-right: [w25] -> _
    shift-left: _ -> [w24]
    shift-right: [w23] -> _
    shift-left: _ -> [w22]
    shift-right: [w12] -> _
    shift-left: _ -> [w11]
    tunnel: w5 -> [_]
    tunnel: w1 -> [w9]
    stop <- w76 stop-if-true
    # "use weights"
    # "units"
    # "config file saved okay"
    # "file saved okay"
    # "trajectory complete"
    # "Is Cubic"
    # "waypoints"
    # "Trajectory Config"
    # "Trajectory"
    n7 = feedback-in #1(w17) -> ()
    n8 = feedback #1() -> (w31:bool)  [unwired: 1 in]
    n9 = First Call?() -> (First Call?: T/F=w29:bool)
    n10 = Not Equal?(x=w17, y=w31) -> (x != y?=w30:bool)
    n11 = Or(x=w30, y=w29) -> (x .or. y?=w28:bool)
    n12 = feedback #2(FALSE ("CreateCmdList")) -> (w100:bool)
    n13 = feedback-in #2("ReadConfigFile") -> ()
    n14 = feedback #3(FALSE ("CreateCmdList")) -> (w39:bool)
    n15 = feedback-in #3("WriteConfigFile") -> ()
    n16 = feedback #4(FALSE ("CreateCmdList")) -> (w103:bool)
    n17 = feedback-in #4("Calculate\nTrajectory") -> ()
    n18 = feedback-in #5("WriteTrajFile") -> ()
    n19 = feedback #5(FALSE ("CreateCmdList")) -> (w105:bool)
    n20 = feedback #6(FALSE ("CreateCmdList")) -> (w21:bool)
    n21 = feedback-in #6("WriteJSONFile") -> ()
    n22 = case shown="True" w28 {
      tunnel: w17 -> [_ w110]
      frame False {
      }
      frame True {
        n23 = Select(t=T12."Enabled" ("Disabled"), s=w110, f=T12."Disabled and Grayed Out" ("Disabled")) -> (s? t:f=w107:T12)
        n24 = property on="WriteConfigFile" class="Bool"("DisabledEnum"=w107) -> ()  [unwired: 2 in, 2 out]
        n25 = property on="WriteTrajFile" class="Bool"("DisabledEnum"=w107) -> ()  [unwired: 2 in, 2 out]
        n26 = property on="WriteJSONFile" class="Bool"("DisabledEnum"=w107) -> ()  [unwired: 2 in, 2 out]
      }
    }
    n27 = Compound Arithmetic op=AND("ReadConfigFile", invert w100) -> (w84:bool)
    n28 = Compound Arithmetic op=AND("WriteConfigFile", invert w39) -> (w32:bool)
    n29 = Compound Arithmetic op=AND("Calculate\nTrajectory", invert w103) -> (w87:bool)
    n30 = Compound Arithmetic op=AND("WriteTrajFile", invert w105) -> (w77:bool)
    n31 = Compound Arithmetic op=AND("WriteJSONFile", invert w21) -> (w18:bool)
    n32 = And(x=w17, y=w77) -> (x .and. y?=w90:bool)
    n33 = And(x=w17, y=w18) -> (x .and. y?=w15:bool)
    n34 = And(x=w17, y=w32) -> (x .and. y?=w33:bool)
    n35 = Select(t=5, s=w33, f=0) -> (s? t:f=w35:i32)
    n36 = Select(t=1, s=w84, f=w35) -> (s? t:f=w85:i32)
    n37 = Select(t=2, s=w87, f=w85) -> (s? t:f=w88:i32)
    n38 = Select(t=3, s=w90, f=w88) -> (s? t:f=w14:i32)
    n39 = Select(t=4, s=w15, f=w14) -> (s? t:f=w13:i32)
    n40 = Select(t=6, s="End Program", f=w13) -> (s? t:f=w83:i32)
    n41 = case shown="0, Default" w83 {
      tunnel: w49 -> [_ w244 w418 w600 w649 w787 w821]
      tunnel: w53 -> [_ w242 w420 w602 w651 w789 w819]
      tunnel: w48 -> [_ w245 w409 w599 w648 w786 w822]
      tunnel: w52 -> [_ w243 w419 w601 w650 w788 w820]
      tunnel: w55 -> [_ w241 w421 w603 w652 w790 w818]
      tunnel: w59 -> [_ w239 w422 w605 w654 w792 w816]
      tunnel: w58 -> [_ w240 w423 w604 w653 w791 w817]
      tunnel: w60 -> [_ w238 w424 w606 w655 w793 w815]
      tunnel: w61 -> [_ w237 w425 w607 w656 w794 w814]
      tunnel: w70 -> [_ w236 w429 w608 w657 w795 w813]
      tunnel: w71 -> [_ w235 w428 w609 w658 w796 w812]
      tunnel: w72 -> [_ w234 w427 w610 w659 w797 w811]
      tunnel: w68 -> [_ w232 w430 w612 w661 w799 w809]
      tunnel: [w180 w222 w413 w617 w665 w801 w830] -> w97
      tunnel: w96 -> [w180 w228 _ w617 w665 w801 w830]
      tunnel: [w179 w221 w414 w616 w664 w781 w829] -> w95
      tunnel: w94 -> [w179 w227 _ w616 w664 w781 w829]
      tunnel: [w178 w220 w412 w615 w663 w780 w828] -> w79
      tunnel: [w119 w223 w406 w592 w642 w782 w831] -> w82
      tunnel: w81 -> [_ w229 w406 w592 w642 w782 w831]
      tunnel: w80 -> [w178 w226 _ w615 w663 w780 w828]
      tunnel: [w177 w219 w437 w614 w662 w800 w827] -> w78
      tunnel: w17 -> [w177 w225 _ w614 w662 w800 w827]
      tunnel: [FALSE FALSE FALSE FALSE FALSE FALSE TRUE] -> w76
      tunnel: [w174 w218 w400 w613 w639 w779 w826] -> w74
      tunnel: w75 -> [w174 w224 _ _ w639 w779 w826]
      tunnel: [w134 w232 w430 w612 w661 w799 w809] -> w73
      tunnel: w69 -> [_ w233 w426 w611 w660 w798 w810]
      tunnel: ["Use Mecanum \nDrive Kinematics\nConstraint" w236 w429 w608 w657 w795 w813] -> w67
      tunnel: [w155 w235 w428 w609 w658 w796 w812] -> w66
      tunnel: [w136 w234 w427 w610 w659 w797 w811] -> w65
      tunnel: [w135 w233 w426 w611 w660 w798 w810] -> w64
      tunnel: [w121 w237 w425 w607 w656 w794 w814] -> w63
      tunnel: ["Use Swerve Drive\nKinematics\nConstraint" w238 w424 w606 w655 w793 w815] -> w62
      tunnel: ["Max Voltage" w240 w423 w604 w653 w791 w817] -> w57
      tunnel: [w133 w239 w422 w605 w654 w792 w816] -> w56
      tunnel: ["Use Diff Drive\nVoltage\nConstraint" w241 w421 w603 w652 w790 w818] -> w54
      tunnel: [w166 w242 w420 w602 w651 w789 w819] -> w51
      tunnel: ["Use Centripetal\nAcceleration\nConstaint" w243 w419 w601 w650 w788 w820] -> w50
      tunnel: [w163 w244 w418 w600 w649 w787 w821] -> w47
      tunnel: ["Use Diff Drive\nKinematic\nConstraint" w245 w409 w599 w648 w786 w822] -> w46
      tunnel: w45 -> [_ w246 w417 w598 w647 w785 w823]
      tunnel: w44 -> [_ w247 w416 w597 w646 w784 w824]
      tunnel: w43 -> [_ w248 w415 w596 w645 w783 w825]
      tunnel: ["Reverse" w246 w417 w598 w647 w785 w823] -> w42
      tunnel: [w160 w247 w416 w597 w646 w784 w824] -> w41
      tunnel: [w159 w248 w415 w596 w645 w783 w825] -> w40
      tunnel: [w158 w213 FALSE ("File Saved\nWithout\nError") w595 w644 w773 w808] -> w27
      tunnel: w26 -> [w158 w212 _ w595 w644 _ w808]
      tunnel: ["Units Selector" w210 w407 w594 w643 w771 w807] -> w25
      tunnel: w24 -> [_ w211 w407 w594 w643 w771 w807]
      tunnel: ["UseWeights" w209 w401 w591 w641 w769 w806] -> w23
      tunnel: w22 -> [_ w208 w401 w591 w641 w769 w806]
      tunnel: [w116 w207 w400 w590 w640 w768 w805] -> w12
      tunnel: w11 -> [w116 w206 _ w590 _ w768 w805]
      tunnel: "Trajectory Type" -> [_ _ _ w589 w638 _ _]
      tunnel: w9 -> [w111 _ _ _ _ _ _]
      frame 0, Default {
        # "Weighted waypoints"
        # "reverse"
        # "robot info"
        # "Diff Drive"
        # "Cent Accel"
        # "Diff Volt"
        # "Swerve Drive"
        # "Mechanum Drive"
        # "Read the User Inputs"
        # "trajectory config"
        # "waypoints"
        # "Default - Read user inputs"
        n42 = call <vilib>:"Translation_GetXY.vi"("In Translation"="Left Rear") -> ("Y"=w144:dbl, "X"=w146:dbl)  [unwired: 9 in]
        n43 = call <vilib>:"Translation_GetXY.vi"("In Translation"="Right Rear") -> ("Y"=w139:dbl, "X"=w141:dbl)  [unwired: 9 in]
        n44 = call <vilib>:"Translation_GetXY.vi"("In Translation"="Right Front") -> ("Y"=w149:dbl, "X"=w151:dbl)  [unwired: 9 in]
        n45 = call <vilib>:"Translation_GetXY.vi"("In Translation"="Left Front") -> ("Y"=w154:dbl, "X"=w157:dbl)  [unwired: 9 in]
        n46 = for {
          tunnel: "Wheels" -> [w201] mode=indexing
          tunnel: [w200] -> w121 mode=indexing
          tunnel: "Units Selector" -> [w199]
          n47 = call <vilib>:"Translation_GetXY.vi"("In Translation"=w201) -> ("Y"=w203:dbl, "X"=w205:dbl)  [unwired: 9 in]
          n48 = call "Create_Trajectory_Units_To_Meters.vi"("Units Selector"=w199, "Units"=w205) -> ("Meters"=w204:dbl)  [unwired: 9 in]
          n49 = call "Create_Trajectory_Units_To_Meters.vi"("Units Selector"=w199, "Units"=w203) -> ("Meters"=w202:dbl)  [unwired: 9 in]
          n50 = call <vilib>:"Translation_Create.vi"("Y"=w202, "X"=w204) -> ("TRANSLATION"=w200:T3)  [unwired: 9 in]
        }
        "Wheels M" <- w121
        n51 = Unbundle By Name("SIMPLE_MOTOR_FF") -> ("Ks"=w131:dbl, "Kv"=w130:dbl, "Ka"=w123:dbl)
        n52 = call "Create_Trajectory_Units_To_Meters.vi"("Units Selector"="Units Selector", "Units"=w146) -> ("Meters"=w145:dbl)  [unwired: 9 in]
        n53 = call "Create_Trajectory_Units_To_Meters.vi"("Units Selector"="Units Selector", "Units"=w141) -> ("Meters"=w140:dbl)  [unwired: 9 in]
        n54 = call "Create_Trajectory_Units_To_Meters.vi"("Units Selector"="Units Selector", "Units"=w151) -> ("Meters"=w150:dbl)  [unwired: 9 in]
        n55 = call "Create_Trajectory_Units_To_Meters.vi"("Units Selector"="Units Selector", "Units"=w157) -> ("Meters"=w156:dbl)  [unwired: 9 in]
        n56 = call "Create_Trajectory_Units_To_Meters.vi"("Units Selector"="Units Selector", "Units"=w144) -> ("Meters"=w143:dbl)  [unwired: 9 in]
        n57 = call "Create_Trajectory_Units_To_Meters.vi"("Units Selector"="Units Selector", "Units"=w139) -> ("Meters"=w138:dbl)  [unwired: 9 in]
        n58 = call "Create_Trajectory_Units_To_Meters.vi"("Units Selector"="Units Selector", "Units"=w149) -> ("Meters"=w148:dbl)  [unwired: 9 in]
        n59 = call "Create_Trajectory_Units_To_Meters.vi"("Units Selector"="Units Selector", "Units"=w154) -> ("Meters"=w153:dbl)  [unwired: 9 in]
        n60 = Reciprocal(x=w130) -> (1/x=w129:dbl)
        n61 = Reciprocal(x=w123) -> (1/x=w126:dbl)
        n62 = call <vilib>:"Translation_Create.vi"("Y"=w143, "X"=w145) -> ("TRANSLATION"=w135:T3)  [unwired: 9 in]
        "Left Rear M" <- w135
        n63 = call <vilib>:"Translation_Create.vi"("Y"=w138, "X"=w140) -> ("TRANSLATION"=w134:T3)  [unwired: 9 in]
        "Right Rear M" <- w134
        n64 = call "Create_Trajectory_Units_To_Meters.vi"("Units Selector"="Units Selector", "Units"=w129) -> ("Meters"=w128:dbl)  [unwired: 9 in]
        n65 = call <vilib>:"Translation_Create.vi"("Y"=w148, "X"=w150) -> ("TRANSLATION"=w136:T3)  [unwired: 9 in]
        "Right Front M" <- w136
        n66 = call <vilib>:"Translation_Create.vi"("Y"=w153, "X"=w156) -> ("TRANSLATION"=w155:T3)  [unwired: 9 in]
        "Left Front M" <- w155
        n67 = call "Create_Trajectory_Units_To_Meters.vi"("Units Selector"="Units Selector", "Units"=w126) -> ("Meters"=w125:dbl)  [unwired: 9 in]
        n68 = feedback-in #7("Field Selector") -> ()
        n69 = feedback #7("ZZZ" ("Field Selector")) -> (w115:string)
        n70 = for {
          tunnel: "WayPoints" -> [w191] mode=indexing
          tunnel: [w190] -> w119 mode=indexing
          tunnel: "Units Selector" -> [w189]
          # "degrees -> radians\nUNITS -> meters\n\nweight unchanged"
          n71 = in-place {
            in-place-border: w189 -> [w192]
            n72 = in-place-cluster #8(w191) -> ("ANGLE"=w193:dbl, "X"=w198:dbl, "Y"=w196:dbl)
            n73 = call <vilib>:"Conv_Deg_Radians.vi"("Degress"=w193) -> ("Radians"=w194:dbl)  [unwired: 10 in]
            n74 = call "Create_Trajectory_Units_To_Meters.vi"("Units Selector"=w192, "Units"=w198) -> ("Meters"=w197:dbl)  [unwired: 9 in]
            n75 = call "Create_Trajectory_Units_To_Meters.vi"("Units Selector"=w192, "Units"=w196) -> ("Meters"=w195:dbl)  [unwired: 9 in]
            n76 = in-place-cluster #8("ANGLE"=w194, "X"=w197, "Y"=w195) -> (w190:T5)
          }
        }
        n77 = Reciprocal(x=w128) -> (1/x=w127:dbl)
        n78 = Reciprocal(x=w125) -> (1/x=w124:dbl)
        n79 = call "Create_Trajectory_Units_To_Meters.vi"("Units Selector"="Units Selector", "Units"="MaxVelocity") -> ("Meters"=w159:dbl)  [unwired: 9 in]
        "MaxVelocity M/S" <- w159
        n80 = Not Equal?(x="Field Selector", y=w115) -> (x != y?=w113:bool)
        n81 = call "Create_Trajectory_Units_To_Meters.vi"("Units Selector"="Units Selector", "Units"="MaxAcceleration") -> ("Meters"=w160:dbl)  [unwired: 9 in]
        "MaxAcceleration M/S^2" <- w160
        n82 = call "Create_Trajectory_Units_To_Meters.vi"("Units Selector"="Units Selector", "Units"="Wheelbase Width") -> ("Meters"=w163:dbl)  [unwired: 9 in]
        "Wheelbase Width M" <- w163
        n83 = call "Create_Trajectory_Units_To_Meters.vi"("Units Selector"="Units Selector", "Units"="Max Cent Accel") -> ("Meters"=w166:dbl)  [unwired: 9 in]
        "Max Cent Accel M/S^2" <- w166
        n84 = call <vilib>:"SimpleMotorFF_New.vi"("Ka"=w124, "Kv"=w127, "Ks"=w131) -> ("SIMPLE_MOTOR_FF"=w133:T4)  [unwired: 8 in]
        "SIMPLE_MOTOR_FF M" <- w133
        n85 = case shown="True" w113 {
          tunnel: "Field Selector" -> [_ w187]
          tunnel: w111 -> [_ w186]
          frame False {
          }
          frame True {
            n86 = call "Create_Trajectory_Get_Field_Info.vi"("Field Selector"=w187) -> ("value"=w188:string, "input cluster"=w185:T25)  [unwired: 9 in]
            n87 = call "Create_Trajectory_Read_Field_Pic.vi"("value"=w188) -> ("Refnum out"=w184:T6)  [unwired: 7 in, 3 out]
            n88 = call "Create_Trajectory_Field_Crop_and_Scale.vi"("Disp Y Size Pixel"=430, "Disp X Size Pixel"=860, "Field Image"=w184, "field Info"=w185, "Display Image"=w186) -> ("Disp Image Out"=→"Field Display":T6)  [unwired: 5 in, 1 out]
          }
        }
        n89 = Wait (ms)(milliseconds to wait=u32 50) -> ()  [unwired: 1 out]
      }
      frame 1 {
        # "Read\nFile"
        # "Read config from trajectory File"
        n90 = call-poly <vilib>:"Read From XML File.vi"("XML File Path"="Read Config File Name") -> ("error out"=w217:errorcluster, "XML Elements"=w230:string)  [unwired: 8 in, 1 out]
        n91 = case shown="No Error" w217 {
          tunnel: w230 -> [w256 _]
          tunnel: w229 -> [w276 w399]
          tunnel: w228 -> [w275 w398]
          tunnel: w227 -> [w274 w397]
          tunnel: w226 -> [w273 w396]
          tunnel: w225 -> [w272 w395]
          tunnel: w224 -> [w271 w394]
          tunnel: [w270 w399] -> w223
          tunnel: [w269 w398] -> w222
          tunnel: [w268 w397] -> w221
          tunnel: [w267 w396] -> w220
          tunnel: [w266 w395] -> w219
          tunnel: [w265 w394] -> w218
          tunnel: w217 -> [w255 w393]
          tunnel: [w263 w393] -> w216
          tunnel: [w262 FALSE] -> w215
          tunnel: [w264 "" ("Write Config File Comment")] -> w214
          tunnel: [w261 w390] -> w213
          tunnel: w212 -> [w260 w390]
          tunnel: w211 -> [w257 w389]
          tunnel: [w259 w389] -> w210
          tunnel: [w253 w388] -> w209
          tunnel: w208 -> [w252 w388]
          tunnel: [w251 w387] -> w207
          tunnel: w206 -> [w250 w387]
          frame No Error {
            # "parse\nXML"
            # "A little bit of a \nkludge to read \nboth v2 and v1\nfile formats...."
            n92 = call "Create_Trajectory_Config_Parse_V1_V2_V3.vi"("error in (no error)"=w255, "Units Selector"=w257, "XML Elements"=w256) -> ("error out"=w258:errorcluster, "TrajCreateConfig"=w254:T14)  [unwired: 7 in]
            n93 = case shown="No Error" w258 {
              tunnel: w276 -> [_ w386]
              tunnel: w275 -> [_ w385]
              tunnel: w274 -> [_ w384]
              tunnel: w273 -> [_ w383]
              tunnel: w272 -> [_ w382]
              tunnel: w271 -> [_ w381]
              tunnel: [w347 w386] -> w270
              tunnel: [T13 {"TotalTImeSecs"=0.0, "States"=[]} ("TRAJECTORY") w385] -> w269
              tunnel: [w346 w384] -> w268
              tunnel: [w348 w383] -> w267
              tunnel: [FALSE w382] -> w266
              tunnel: [FALSE ("File Saved\nWithout\nError") w381] -> w265
              tunnel: w254 -> [w353 _]
              tunnel: [w325 "" ("Write Config File Comment")] -> w264
              tunnel: w258 -> [w351 w379]
              tunnel: [w351 w379] -> w263
              tunnel: [TRUE FALSE] -> w262
              tunnel: [FALSE ("File Saved\nWithout\nError") w377] -> w261
              tunnel: w260 -> [_ w377]
              tunnel: w257 -> [_ w376]
              tunnel: [w284 w376] -> w259
              tunnel: [w281 w375] -> w253
              tunnel: w252 -> [_ w375]
              tunnel: [FALSE ("File Saved\nWithout\nError") w374] -> w251
              tunnel: w250 -> [_ w374]
              frame No Error {
                # "This really doesn't do much\nstate 1 will write over this from\nthe user inputs....."
                # "Write to local\nuser controls"
                # "not used"
                # "not used"
                # "should make this a subvi"
                n94 = Unbundle By Name(w353) -> ("Write Config File Name"=w278:path, "Write Config File Comment"=w325:string, "WayPoints"=w347:T5[], "TRAJECTORY_CONFIG"=w346:T15, "IsCubic"=w348:bool, "Units Selector"=w284:T2, "UseWeights"=w281:bool)
                n95 = Unbundle By Name(w346) -> ("MaxVelocity"=w343:dbl, "Max Acceleration"=w342:dbl, "Reversed"=w341:bool, "DiffDrKineConstntDefined"=w340:bool, "CentAcellConstntDefined"=w339:bool, "DiffDrVoltConstntDefined"=w338:bool, "SwerveDrKineConstntDefined"=w337:bool, "MecanumDrKineConstntDefined"=w336:bool, "DIFF_DRIVE_KINE_CONSTRAINT"=w335:T16, "CENTRIPETAL_ACCEL_CONSTRAINT"=w332:T18, "DIFF_DRIVE_VOLTAGE_CONSTRAINT"=w329:T22, "MECANUM_DRIVE_KINE_CONSTRAINT"=w327:T23, "SWERVE_DRIVE_KINE_CONSTRAINT"=w326:T19)  [unwired: 2 out]
                n96 = Unbundle By Name(w327) -> ("MECA_DRIVE_KINEMATICS.FrontLeft"=w300:T3, "MECA_DRIVE_KINEMATICS.FrontRight"=w301:T3, "MECA_DRIVE_KINEMATICS.RearLeft"=w302:T3, "MECA_DRIVE_KINEMATICS.RearRight"=w303:T3)
                n97 = Unbundle By Name(w335) -> ("DIFF_DRIVE_KINEMATICS.TrackWidth_Meters"=w333:dbl)
                n98 = Unbundle By Name(w332) -> ("Max Cent Accel"=w330:dbl)
                n99 = Unbundle By Name(w329) -> ("Max Voltage"=w328:dbl, "SIMPLE_MOTOR_FF"=w286:T4)
                n100 = Unbundle By Name(w326) -> ("SwerveKinematics.Modules"=w320:T3[])
                n101 = Unbundle By Name(w286) -> ("Ks"=w295:dbl, "Kv"=w294:dbl, "Ka"=w287:dbl)
                n102 = for {
                  tunnel: w347 -> [w364] mode=indexing
                  tunnel: [w363] -> w283 mode=indexing
                  tunnel: w284 -> [w362]
                  # "radians -> degrees\nmeters -> inches\nWeights stay the same"
                  n103 = in-place {
                    in-place-border: w362 -> [w365]
                    n104 = in-place-cluster #9(w364) -> ("ANGLE"=w366:dbl, "X"=w371:dbl, "Y"=w369:dbl)
                    n105 = call "Create_Trajectory_Meters_To_Units.vi"("Units Selector"=w365, "Meters"=w369) -> ("Units"=w368:dbl)  [unwired: 9 in]
                    n106 = call <vilib>:"Conv_Radians_Deg.vi"("Radians"=w366) -> ("Degrees"=w367:dbl)  [unwired: 10 in]
                    n107 = call "Create_Trajectory_Meters_To_Units.vi"("Units Selector"=w365, "Meters"=w371) -> ("Units"=w370:dbl)  [unwired: 9 in]
                    n108 = in-place-cluster #9("ANGLE"=w367, "X"=w370, "Y"=w368) -> (w363:T5)
                  }
                }
                n109 = case shown="True" w348 {
                  tunnel: [enum32{"Radio Selection 1", "Radio Selection 2"}."Radio Selection 2" ("Spline Type") enum32{"Radio Selection 1", "Radio Selection 2"}."Radio Selection 1" ("Spline Type")] -> w349
                  frame False {
                  }
                  frame True {
                  }
                }
                n110 = Reciprocal(x=w294) -> (1/x=w293:dbl)
                n111 = Reciprocal(x=w287) -> (1/x=w290:dbl)
                n112 = call "ChangeFileExtension.vi"("NewExtenion"=".json", "In FileName"=w278) -> ("Out FileName"=w277:path)  [unwired: 9 in]
                n113 = call "ChangeFileExtension.vi"("NewExtenion"=".csv", "In FileName"=w278) -> ("Out FileName"=w324:path)  [unwired: 9 in]
                n114 = call <vilib>:"Translation_GetXY.vi"("In Translation"=w300) -> ("Y"=w317:dbl, "X"=w319:dbl)  [unwired: 9 in]
                n115 = call <vilib>:"Translation_GetXY.vi"("In Translation"=w301) -> ("Y"=w313:dbl, "X"=w315:dbl)  [unwired: 9 in]
                n116 = call <vilib>:"Translation_GetXY.vi"("In Translation"=w302) -> ("Y"=w309:dbl, "X"=w311:dbl)  [unwired: 9 in]
                n117 = for {
                  tunnel: w320 -> [w357] mode=indexing
                  tunnel: [w356] -> w321 mode=indexing
                  tunnel: w284 -> [w355]
                  n118 = call <vilib>:"Translation_GetXY.vi"("In Translation"=w357) -> ("Y"=w359:dbl, "X"=w361:dbl)  [unwired: 9 in]
                  n119 = call "Create_Trajectory_Meters_To_Units.vi"("Units Selector"=w355, "Meters"=w361) -> ("Units"=w360:dbl)  [unwired: 9 in]
                  n120 = call "Create_Trajectory_Meters_To_Units.vi"("Units Selector"=w355, "Meters"=w359) -> ("Units"=w358:dbl)  [unwired: 9 in]
                  n121 = call <vilib>:"Translation_Create.vi"("Y"=w358, "X"=w360) -> ("TRANSLATION"=w356:T3)  [unwired: 9 in]
                }
                n122 = call <vilib>:"Translation_GetXY.vi"("In Translation"=w303) -> ("Y"=w305:dbl, "X"=w307:dbl)  [unwired: 9 in]
                n123 = call "Create_Trajectory_Meters_To_Units.vi"("Units Selector"=w284, "Meters"=w293) -> ("Units"=w292:dbl)  [unwired: 9 in]
                n124 = call "Create_Trajectory_Meters_To_Units.vi"("Units Selector"=w284, "Meters"=w343) -> ("Units"=w344:dbl)  [unwired: 9 in]
                n125 = call "Create_Trajectory_Meters_To_Units.vi"("Units Selector"=w284, "Meters"=w290) -> ("Units"=w289:dbl)  [unwired: 9 in]
                n126 = local write "Trajectory JSON File Name"(w277) -> ()
                n127 = local write "Trajectory CSV File Name"(w324) -> ()
                n128 = call "Create_Trajectory_Meters_To_Units.vi"("Units Selector"=w284, "Meters"=w319) -> ("Units"=w318:dbl)  [unwired: 9 in]
                n129 = call "Create_Trajectory_Meters_To_Units.vi"("Units Selector"=w284, "Meters"=w342) -> ("Units"=w345:dbl)  [unwired: 9 in]
                n130 = call "Create_Trajectory_Meters_To_Units.vi"("Units Selector"=w284, "Meters"=w315) -> ("Units"=w314:dbl)  [unwired: 9 in]
                n131 = local write "Units Selector"(w284) -> ()
                n132 = local write "UseWeights"(w281) -> ()
                n133 = local write "Write Config File Name"(w278) -> ()
                n134 = local write "Write Config File Comment"(w325) -> ()
                n135 = local write "Trajectory File Comment"(w325) -> ()
                n136 = call "Create_Trajectory_Meters_To_Units.vi"("Units Selector"=w284, "Meters"=w311) -> ("Units"=w310:dbl)  [unwired: 9 in]
                n137 = Reciprocal(x=w292) -> (1/x=w291:dbl)
                n138 = call "Create_Trajectory_Meters_To_Units.vi"("Units Selector"=w284, "Meters"=w307) -> ("Units"=w306:dbl)  [unwired: 9 in]
                n139 = Reciprocal(x=w289) -> (1/x=w288:dbl)
                n140 = call "Create_Trajectory_Meters_To_Units.vi"("Units Selector"=w284, "Meters"=w317) -> ("Units"=w316:dbl)  [unwired: 9 in]
                n141 = call "Create_Trajectory_Meters_To_Units.vi"("Units Selector"=w284, "Meters"=w313) -> ("Units"=w312:dbl)  [unwired: 9 in]
                n142 = local write "Use Mecanum \nDrive Kinematics\nConstraint"(w336) -> ()
                n143 = call "Create_Trajectory_Meters_To_Units.vi"("Units Selector"=w284, "Meters"=w309) -> ("Units"=w308:dbl)  [unwired: 9 in]
                n144 = call "Create_Trajectory_Meters_To_Units.vi"("Units Selector"=w284, "Meters"=w305) -> ("Units"=w304:dbl)  [unwired: 9 in]
                n145 = call "Create_Trajectory_Meters_To_Units.vi"("Units Selector"=w284, "Meters"=w333) -> ("Units"=w334:dbl)  [unwired: 9 in]
                n146 = call "Create_Trajectory_Meters_To_Units.vi"("Units Selector"=w284, "Meters"=w330) -> ("Units"=w331:dbl)  [unwired: 9 in]
                n147 = local write "Use Swerve Drive\nKinematics\nConstraint"(w337) -> ()
                n148 = local write "Use Centripetal\nAcceleration\nConstaint"(w339) -> ()
                n149 = call <vilib>:"SimpleMotorFF_New.vi"("Ka"=w288, "Kv"=w291, "Ks"=w295) -> ("SIMPLE_MOTOR_FF"=w285:T4)  [unwired: 8 in]
                n150 = local write "Use Diff Drive\nKinematic\nConstraint"(w340) -> ()
                n151 = local write "MaxVelocity"(w344) -> ()
                n152 = local write "MaxAcceleration"(w345) -> ()
                n153 = local write "Spline Type"(w349) -> ()
                n154 = call <vilib>:"Translation_Create.vi"("Y"=w316, "X"=w318) -> ("TRANSLATION"=w299:T3)  [unwired: 9 in]
                n155 = local write "Use Diff Drive\nVoltage\nConstraint"(w338) -> ()
                n156 = call <vilib>:"Translation_Create.vi"("Y"=w312, "X"=w314) -> ("TRANSLATION"=w298:T3)  [unwired: 9 in]
                n157 = call <vilib>:"Translation_Create.vi"("Y"=w308, "X"=w310) -> ("TRANSLATION"=w297:T3)  [unwired: 9 in]
                n158 = call <vilib>:"Translation_Create.vi"("Y"=w304, "X"=w306) -> ("TRANSLATION"=w296:T3)  [unwired: 9 in]
                n159 = local write "Reverse"(w341) -> ()
                n160 = local write "Wheelbase Width"(w334) -> ()
                n161 = local write "Max Cent Accel"(w331) -> ()
                n162 = local write "SIMPLE_MOTOR_FF"(w285) -> ()
                n163 = local write "Max Voltage"(w328) -> ()
                n164 = local write "WayPoints"(w283) -> ()
                n165 = local write "Left Front"(w299) -> ()
                n166 = local write "Right Front"(w298) -> ()
                n167 = local write "Right Rear"(w296) -> ()
                n168 = local write "Left Rear"(w297) -> ()
                n169 = local write "Wheels"(w321) -> ()
              }
              frame Error {
              }
            }
          }
          frame Error {
          }
        }
        "Config File Read\nWithout Error" <- w215
        "Config File  Read Error" <- w216
        "Read Config File Comment" <- w214
      }
      frame 2 {
        w400 = FALSE ("File Saved\nWithout\nError")
        # "#TODO  If differential speed is exceeded, flag an error."
        # "Waypoints"
        # "diff max speed\nexceeded."
        # "Inches/Sec"
        # "Inches"
        # "Input was Inches, plot inches...."
        # "max velocity"
        # "Create Trajectory"
        # "allow a little excess"
        # "in meters"
        # "Diff drive"
        # "Distance\nVelocity\nAcceleration\nRotatonal Velocity\nHeading\nJerk (Delta Accel)"
        # "FIELD POSITION\nGRAPH"
        # "GRAPH OF DATA"
        # "construct the trajectory\nconfiguration information"
        # "trajectory \nmeters, radians"
        # "DIFFERENTIAL DRIVE MAX SPEED"
        # "Create absolute Trajectory\nStates"
        n170 = call <vilib>:"TrajectoryConfig_Create.vi"("MaxAcceleration"=w416, "MaxVelocity"=w415) -> ("TRAJECTORY_CONFIG"=w432:T15)  [unwired: 9 in]
        n171 = call <vilib>:"TrajectoryConfig_setReversed.vi"("Reversed"=w417, "inTRAJECTORY_CONFIG"=w432) -> ("outTRAJECTORY_CONFIG"=w431:T15)  [unwired: 9 in]
        n172 = call <vilib>:"DiffKinematics_New.vi"("TrackWidth_Meters"=w418) -> ("DIFF_DRIVE_KINEMATICS"=w445:T17)  [unwired: 10 in]
        n173 = case shown="True" w409 {
          tunnel: w431 -> [w576 w579]
          tunnel: [w576 w578] -> w473
          tunnel: w445 -> [_ w577]
          frame False {
          }
          frame True {
            n174 = call <vilib>:"TrajectoryConfig_setKinematicsDiffDrive.vi"("DIFF_DRIVE_KINEMATICS"=w577, "inTRAJECTORY_CONFIG"=w579) -> ("outTRAJECTORY_CONFIG"=w578:T15)  [unwired: 9 in]
          }
        }
        n175 = for {
          tunnel: w406 -> [w487] mode=indexing
          tunnel: [w484] -> w405 mode=indexing
          tunnel: [w483] -> w404 mode=indexing
          n176 = Unbundle By Name(w487) -> ("X"=w486:dbl, "Y"=w485:dbl)
          n177 = call <vilib>:"Conv_Meters_Inches.vi"("Meters"=w486) -> ("Inches"=w484:dbl)  [unwired: 10 in]
          n178 = call <vilib>:"Conv_Meters_Inches.vi"("Meters"=w485) -> ("Inches"=w483:dbl)  [unwired: 10 in]
        }
        n179 = case shown="True" w419 {
          tunnel: w473 -> [w572 w575]
          tunnel: w420 -> [_ w574]
          tunnel: [w572 w573] -> w453
          frame False {
          }
          frame True {
            n180 = call <vilib>:"TrajectoryConfig_setCentripetalAccel.vi"("Max Cent Accel"=w574, "inTRAJECTORY_CONFIG"=w575) -> ("outTRAJECTORY_CONFIG"=w573:T15)  [unwired: 9 in]
          }
        }
        n181 = case shown="True" w421 {
          tunnel: w453 -> [w530 w536]
          tunnel: [w530 w535] -> w452
          tunnel: w422 -> [_ w534]
          tunnel: w418 -> [_ w533]
          tunnel: w423 -> [_ w531]
          frame False {
          }
          frame True {
            n182 = call <vilib>:"DiffKinematics_New.vi"("TrackWidth_Meters"=w533) -> ("DIFF_DRIVE_KINEMATICS"=w532:T17)  [unwired: 10 in]
            n183 = call <vilib>:"TrajectoryConfig_setVoltageDiffDrive.vi"("SIMPLE_MOTOR_FF"=w534, "DIFF_DRIVE_KINEMATICS"=w532, "Max Voltage"=w531, "inTRAJECTORY_CONFIG"=w536) -> ("outTRAJECTORY_CONFIG"=w535:T15)  [unwired: 7 in]
          }
        }
        n184 = case shown="True" w424 {
          tunnel: [w525 w529] -> w441
          tunnel: w452 -> [w525 w528]
          tunnel: w425 -> [_ w526]
          frame False {
          }
          frame True {
            n185 = call <vilib>:"SwerveKinematics_NewX.vi"("Wheels"=w526) -> ("SWERVE_DRIVE_KINEMATICS"=w527:T20)  [unwired: 10 in]
            n186 = call <vilib>:"TrajectoryConfig_setKinematicsSwerveDrive.vi"("SWERVE_DRIVE_KINEMATICS"=w527, "inTRAJECTORY_CONFIG"=w528) -> ("outTRAJECTORY_CONFIG"=w529:T15)  [unwired: 9 in]
          }
        }
        n187 = case shown="True" w429 {
          tunnel: [w488 w495] -> w414
          tunnel: w441 -> [w488 w494]
          tunnel: w428 -> [_ w492]
          tunnel: w427 -> [_ w491]
          tunnel: w426 -> [_ w490]
          tunnel: w430 -> [_ w489]
          frame False {
          }
          frame True {
            n188 = call <vilib>:"MecaKinematics_New.vi"("RearRight"=w489, "RearLeft"=w490, "FrontRight"=w491, "FrontLeft"=w492) -> ("MECA_DRIVE_KINEMATICS"=w493:T24)  [unwired: 7 in]
            n189 = call <vilib>:"TrajectoryConfig_setKinematicsMecanumDrive.vi"("MECA_DRIVE_KINEMATICS"=w493, "inTRAJECTORY_CONFIG"=w494) -> ("outTRAJECTORY_CONFIG"=w495:T15)  [unwired: 9 in]
          }
        }
        n190 = case shown="\"Radio Selection 1\", Default" "Spline Type" {
          tunnel: [w548 w557] -> w438
          tunnel: w414 -> [w547 w554]
          tunnel: [w549 w556] -> w413
          tunnel: [TRUE FALSE] -> w412
          tunnel: w406 -> [w545 w552]
          tunnel: w401 -> [w539 w550]
          frame "Radio Selection 1", Default {
            # "format\nwaypoints for\nspline functions"
            # "Calc\ncubic\nsplines"
            n191 = call <vilib>:"Util_WeightedWaypoint_To_WeightedWayPoint.vi"("Util_WeightedWayPoints"=w545) -> ("WeightedWayPoints"=w544:T26[])  [unwired: 10 in]
            n192 = call <vilib>:"SplineHelp_GetCubicCtrlVectorsFromWeightedWayPts.vi"("Use Weights"=w539, "WeightedWayPoints"=w544) -> ("Interior WAYPOINTS"=w543:T3[], "SplineControlVectors"=w542:T27[])  [unwired: 8 in]
            n193 = Index Array(array=w542, index #1=0 ("index"), index #2=1 ("index")) -> (element #1=w541:T27, element #2=w540:T27)
            n194 = call <vilib>:"TrajectoryGenerate_Make_Cubic_CtrlVect.vi"("traj_config"=w547, "end-Spline_Ctrl_Vector"=w540, "Interior WAYPOINTS"=w543, "initial-Spline_Ctrl_Vector"=w541) -> ("error out"=w548:errorcluster, "TRAJECTORY"=w549:T13)  [unwired: 6 in]
          }
          frame "Radio Selection 2" {
            # "format\nwaypoints for\nspline functions"
            # "CALC\nQUINTIC\nSPLINE"
            n195 = call <vilib>:"Util_WeightedWaypoint_To_WeightedWayPoint.vi"("Util_WeightedWayPoints"=w552) -> ("WeightedWayPoints"=w551:T26[])  [unwired: 10 in]
            n196 = call <vilib>:"SplineHelp_GetQuinticCtrlVectorsFromWeightedWayPts.vi"("Use Weights"=w550, "WayPoints"=w551) -> ("SplineControlVectors"=w553:T27[])  [unwired: 9 in]
            n197 = call <vilib>:"TrajectoryGenerate_Make_Quintic_CtrlVect.vi"("traj_config"=w554, "input_ControlVectors"=w553) -> ("error out"=w557:errorcluster, "TRAJECTORY"=w556:T13)  [unwired: 8 in]
          }
        }
        "Trajectory calculation error" <- w438
        n198 = Unbundle By Name(w413) -> ("States"=w444:T7[], "TotalTImeSecs"=w448:dbl)
        "Trajectory States" <- w444
        n199 = while {
          tunnel: [w517] -> w450 mode=indexing
          tunnel: [w508] -> w469 mode=indexing
          tunnel: [w510] -> w468 mode=indexing
          tunnel: [w514] -> w467 mode=indexing
          tunnel: [w509] -> w466 mode=indexing
          tunnel: [w524] -> w465 mode=indexing
          shift-right: [w518] -> _
          shift-left: 0.0 -> [w508]
          tunnel: [w512] -> w449 mode=indexing
          tunnel: w448 -> [w504]
          tunnel: w413 -> [w496]
          i -> [w502]
          stop <- w503 stop-if-true
          # "Time Df"
          # "Jerk"
          # "Dist"
          n200 = To Double Precision Float(number=w502) -> (double precision float=w501:dbl)
          n201 = Multiply(x=w501, y=0.02) -> (x*y=w499:dbl)
          n202 = feedback #10(0.0 ("TimeSeconds")) -> (w520:dbl)
          n203 = feedback #11(0.0 ("TimeSeconds")) -> (w522:dbl)
          n204 = feedback #12(0.0 ("TimeSeconds")) -> (w515:dbl)
          n205 = call <vilib>:"Trajectory_Sample.vi"("Time"=w499, "InputTRAJECTORY"=w496) -> ("OutputTRAJ_STATE"=w497:T7)  [unwired: 9 in]
          n206 = call <vilib>:"Util_TrajectoryState_Meters_To_Inches.vi"("absTRAJECTORY"=w497) -> ("outputRelativeTRAJECTORY"=w498:T7)  [unwired: 10 in]
          n207 = Unbundle By Name(w498) -> ("TimeSeconds"=w517:dbl, "Velocity"=w510:dbl, "Acceleration"=w514:dbl, "Curvature"=w511:dbl, "POSE.ROTATION.VALUE"=w524:dbl)
          n208 = feedback-in #10(w510) -> ()
          n209 = feedback-in #11(w517) -> ()
          n210 = feedback-in #12(w514) -> ()
          n211 = Add(x=w510, y=w520) -> (x+y=w519:dbl)
          n212 = Subtract(x=w517, y=w522) -> (x-y=w505:dbl)
          n213 = Subtract(x=w514, y=w515) -> (x-y=w513:dbl)
          n214 = Compound Arithmetic op=MULTIPLY(w519, 0.5 ("value"), w505) -> (w507:dbl)
          n215 = Divide(x=w513, y=w505) -> (x/y=w512:dbl)
          n216 = Add(x=w507, y=w508) -> (x+y=w518:dbl)
          n217 = Greater Or Equal?(x=w499, y=w504) -> (x >= y?=w503:bool)
          n218 = Multiply(x=w510, y=w511) -> (x*y=w509:dbl)
        }
        n219 = for {
          tunnel: w444 -> [w562] mode=indexing
          tunnel: w418 -> [w571]
          tunnel: [w569] -> w460 mode=indexing
          tunnel: [w568] -> w459 mode=indexing
          tunnel: [w565] -> w458 mode=indexing
          tunnel: [w563] -> w457 mode=indexing
          tunnel: [w559] -> w447 mode=indexing
          tunnel: [w558] -> w446 mode=indexing
          n220 = Unbundle By Name(w562) -> ("POSE.TRANSLATION.X"=w561:dbl, "POSE.TRANSLATION.Y"=w560:dbl)
          n221 = call <vilib>:"Util_TrajState_to_DiffDrive_WheelPos.vi"("Wheelbase"=w571, "TRAJ_STATE"=w562) -> ("Right Y"=w564:dbl, "Right X"=w566:dbl, "Left Y"=w567:dbl, "Left X"=w570:dbl)  [unwired: 6 in]
          n222 = call <vilib>:"Conv_Meters_Inches.vi"("Meters"=w570) -> ("Inches"=w569:dbl)  [unwired: 10 in]
          n223 = call <vilib>:"Conv_Meters_Inches.vi"("Meters"=w566) -> ("Inches"=w565:dbl)  [unwired: 10 in]
          n224 = call <vilib>:"Conv_Meters_Inches.vi"("Meters"=w561) -> ("Inches"=w558:dbl)  [unwired: 10 in]
          n225 = call <vilib>:"Conv_Meters_Inches.vi"("Meters"=w567) -> ("Inches"=w568:dbl)  [unwired: 10 in]
          n226 = call <vilib>:"Conv_Meters_Inches.vi"("Meters"=w564) -> ("Inches"=w563:dbl)  [unwired: 10 in]
          n227 = call <vilib>:"Conv_Meters_Inches.vi"("Meters"=w560) -> ("Inches"=w559:dbl)  [unwired: 10 in]
        }
        n228 = for {
          tunnel: [w581] -> w480 mode=indexing
          tunnel: [w580] -> w478 mode=indexing
          tunnel: w444 -> [w588] mode=indexing
          tunnel: w445 -> [w582]
          # "see if max speed violated  by\neither wheel speed"
          n229 = Unbundle By Name(w588) -> ("Velocity"=w586:dbl, "Curvature"=w587:dbl)
          n230 = Multiply(x=w586, y=w587) -> (x*y=w584:dbl)
          n231 = call <vilib>:"ChassisSpeeds_New.vi"("vAngular"=w584, "vY"=0.0, "vX"=w586) -> ("CHASSIS"=w583:T28)  [unwired: 8 in]
          n232 = call <vilib>:"DiffKinematics_toWheelSpeed.vi"("CHASSIS Speed"=w583, "DIFF_DRIVE_KINEMATICS"=w582) -> ("RightVelocity"=w580:dbl, "LeftVelocity"=w581:dbl)  [unwired: 8 in]
        }
        n233 = Bundle(w405, w404) -> (w403:cluster{dbl[], dbl[]})  [unwired: 1 in]
        n234 = Bundle(w446, w447) -> (w455:cluster{dbl[], dbl[]})  [unwired: 1 in]
        n235 = Bundle(w460, w459) -> (w454:cluster{dbl[], dbl[]})  [unwired: 1 in]
        n236 = Bundle(w458, w457) -> (w456:cluster{dbl[], dbl[]})  [unwired: 1 in]
        n237 = Absolute Value(x=w480) -> (abs(x)=w479:dbl[])
        n238 = Absolute Value(x=w478) -> (abs(x)=w477:dbl[])
        n239 = Multiply(x=w415, y=1.01) -> (x*y=w439:dbl)
        n240 = Build Array(w455, w454, w456, w403) -> (→"Position":cluster{dbl[], dbl[]}[])
        n241 = Array Max & Min(array=w479) -> (max value=w475:dbl)  [unwired: 3 out]
        n242 = Array Max & Min(array=w477) -> (max value=w474:dbl)  [unwired: 3 out]
        n243 = Greater?(x=w475, y=w439) -> (0:w481:bool)
        n244 = Greater?(x=w474, y=w439) -> (0:w476:bool)
        n245 = Max & Min(x=w475, y=w474) -> (max(x,y)=w443:dbl)  [unwired: 1 out]
        n246 = Bundle(w450, w466) -> (w464:cluster{dbl[], dbl[]})  [unwired: 1 in]
        n247 = Bundle(w450, w465) -> (w463:cluster{dbl[], dbl[]})  [unwired: 1 in]
        n248 = Bundle(w450, w468) -> (w471:cluster{dbl[], dbl[]})  [unwired: 1 in]
        n249 = Bundle(w450, w449) -> (w451:cluster{dbl[], dbl[]})  [unwired: 1 in]
        n250 = Bundle(w450, w469) -> (w472:cluster{dbl[], dbl[]})  [unwired: 1 in]
        n251 = Bundle(w450, w467) -> (w470:cluster{dbl[], dbl[]})  [unwired: 1 in]
        n252 = Compound Arithmetic op=OR(w481, w476) -> (w410:bool)
        n253 = call <vilib>:"Conv_Meters_Inches.vi"("Meters"=w443) -> ("Inches"=→"differential \ndrive \nmax speed":dbl)  [unwired: 10 in]
        n254 = Array Size(array=w444) -> (size(s)=w436:i32)
        "Traj States\nSize" <- w436
        n255 = Build Array(w472, w471, w470, w464, w463, w451) -> (→"Trajectory Data":cluster{dbl[], dbl[]}[])
        n256 = And(x=w410, y=w409) -> (x .and. y?=w408:bool)
        n257 = Not(x=w408) -> (.not. x?=w434:bool)
        n258 = Greater Than 0?(x=w436) -> (x > 0?=w435:bool)
        n259 = And(x=w435, y=w434) -> (x .and. y?=w437:bool)
      }
      frame 3 {
        # "Write trajectory to CSV File"
        n260 = case shown="\"Radio Selection 1\", Default" w589 {
          tunnel: w617 -> [w627 w629]
          tunnel: [w626 w629] -> w621
          tunnel: [TRUE FALSE] -> w619
          frame "Radio Selection 1", Default {
            # "Relative"
            n261 = call <vilib>:"Util_Trajectory_Absolute_To_Relative.vi"("absTRAJECTORY"=w627) -> ("outputRelativeTRAJECTORY"=w626:T13)  [unwired: 10 in]
          }
          frame "Radio Selection 2" {
            # "Absolute"
          }
        }
        n262 = call <vilib>:"Util_Trajectory_WriteFile.vi"("Trajectory is Cubic"=w615, "UseWeights"=w591, "Trajectory Is Relative"=w619, "TRAJECTORY_CONFIG"=w616, "UtilityWayPoints"=w592, "TRAJECTORY"=w621, "Comment"="Trajectory File Comment", "Trajectory File Name"="Trajectory CSV File Name") -> ("error out"=w620:errorcluster)  [unwired: 3 in]
        "Write Trajectory\nFile Error" <- w620
        n263 = local write "Write Config File Comment"("Trajectory File Comment") -> ()
        n264 = case shown="Error .." w620 {
          tunnel: [TRUE ("File Saved\nWithout\nError") FALSE ("File Saved\nWithout\nError")] -> w613
          frame No Error {
          }
          frame Error {
          }
        }
      }
      frame 4 {
        # "Write trajectory to JSON File"
        n265 = case shown="\"Radio Selection 1\", Default" w638 {
          tunnel: w665 -> [w765 w767]
          tunnel: [w764 w767] -> w634
          tunnel: [TRUE FALSE] -> _
          frame "Radio Selection 1", Default {
            # "Relative"
            n266 = call <vilib>:"Util_Trajectory_Absolute_To_Relative.vi"("absTRAJECTORY"=w765) -> ("outputRelativeTRAJECTORY"=w764:T13)  [unwired: 10 in]
          }
          frame "Radio Selection 2" {
            # "Absolute"
          }
        }
        n267 = Unbundle By Name(w634) -> ("States"=w633:T7[])
        n268 = case shown="\"Radio Selection 1\"" "PathWeaver Length Units" {
          tunnel: w633 -> [w667 w668 w692 w722 w742]
          tunnel: [w667 w669 w691 w721 w741] -> w630
          frame "Radio Selection 1" {
            # "Meters - do nothing"
          }
          frame "Radio Selection 2" {
            # "Conv Meters to Centimeters"
            n269 = for {
              tunnel: w668 -> [w671] mode=indexing
              tunnel: [w670] -> w669 mode=indexing
              n270 = in-place {
                n271 = in-place-cluster #13(w671) -> ("Acceleration"=w682:dbl, "TimeSeconds"=w690:dbl, "Velocity"=w680:dbl, "Curvature"=w685:dbl, "POSE.TRANSLATION.X"=w672:dbl, "POSE.TRANSLATION.Y"=w676:dbl, "POSE.ROTATION.VALUE"=w687:dbl, "POSE.ROTATION.COS"=w689:dbl, "POSE.ROTATION.SIN"=w688:dbl)
                n272 = Multiply(x=w672, y=100.0) -> (x*y=w673:dbl)
                n273 = Multiply(x=w676, y=100.0) -> (x*y=w675:dbl)
                n274 = Multiply(x=w680, y=100.0) -> (x*y=w679:dbl)
                n275 = Multiply(x=w682, y=100.0) -> (x*y=w683:dbl)
                n276 = Divide(x=w685, y=100.0 ("Centimeter")) -> (x/y=w686:dbl)
                n277 = in-place-cluster #13("Acceleration"=w683, "TimeSeconds"=w690, "Velocity"=w679, "Curvature"=w686, "POSE.TRANSLATION.X"=w673, "POSE.TRANSLATION.Y"=w675, "POSE.ROTATION.VALUE"=w687, "POSE.ROTATION.COS"=w689, "POSE.ROTATION.SIN"=w688) -> (w670:T7)
              }
            }
          }
          frame "Radio Selection 3" {
            # "Who uses yards ????"
            # "Conv Meters to Yards"
            n278 = for {
              tunnel: w692 -> [w694] mode=indexing
              tunnel: [w693] -> w691 mode=indexing
              n279 = in-place {
                n280 = in-place-cluster #14(w694) -> ("Acceleration"=w714:dbl, "TimeSeconds"=w720:dbl, "Velocity"=w715:dbl, "Curvature"=w712:dbl, "POSE.TRANSLATION.X"=w716:dbl, "POSE.TRANSLATION.Y"=w717:dbl, "POSE.ROTATION.VALUE"=w713:dbl, "POSE.ROTATION.COS"=w719:dbl, "POSE.ROTATION.SIN"=w718:dbl)
                n281 = call <vilib>:"Conv_Meters_Feet.vi"("Meters"=w717) -> ("Feet"=w699:dbl)  [unwired: 10 in]
                n282 = call <vilib>:"Conv_Meters_Feet.vi"("Meters"=w714) -> ("Feet"=w709:dbl)  [unwired: 10 in]
                n283 = call <vilib>:"Conv_Meters_Feet.vi"("Meters"=w715) -> ("Feet"=w705:dbl)  [unwired: 10 in]
                n284 = call <vilib>:"Conv_Meters_Feet.vi"("Meters"=w716) -> ("Feet"=w696:dbl)  [unwired: 10 in]
                n285 = Divide(x=w696, y=3.0) -> (x/y=w695:dbl)
                n286 = Divide(x=w699, y=3.0) -> (x/y=w698:dbl)
                n287 = Divide(x=w709, y=3.0) -> (x/y=w707:dbl)
                n288 = Divide(x=w705, y=3.0) -> (x/y=w704:dbl)
                n289 = call <vilib>:"Conv_Meters_Feet.vi"("Meters"=1.0 ("Centimeter")) -> ("Feet"=w701:dbl)  [unwired: 10 in]
                n290 = Divide(x=w701, y=3.0) -> (x/y=w702:dbl)
                n291 = Divide(x=w712, y=w702) -> (x/y=w711:dbl)
                n292 = in-place-cluster #14("Acceleration"=w707, "TimeSeconds"=w720, "Velocity"=w704, "Curvature"=w711, "POSE.TRANSLATION.X"=w695, "POSE.TRANSLATION.Y"=w698, "POSE.ROTATION.VALUE"=w713, "POSE.ROTATION.COS"=w719, "POSE.ROTATION.SIN"=w718) -> (w693:T7)
              }
            }
          }
          frame "Radio Selection 4" {
            # "Meters Conv to Feet"
            n293 = for {
              tunnel: w722 -> [w724] mode=indexing
              tunnel: [w723] -> w721 mode=indexing
              n294 = in-place {
                n295 = in-place-cluster #15(w724) -> ("Acceleration"=w732:dbl, "TimeSeconds"=w740:dbl, "Velocity"=w734:dbl, "Curvature"=w726:dbl, "POSE.TRANSLATION.X"=w736:dbl, "POSE.TRANSLATION.Y"=w737:dbl, "POSE.ROTATION.VALUE"=w729:dbl, "POSE.ROTATION.COS"=w739:dbl, "POSE.ROTATION.SIN"=w738:dbl)
                n296 = call <vilib>:"Conv_Meters_Feet.vi"("Meters"=w732) -> ("Feet"=w731:dbl)  [unwired: 10 in]
                n297 = call <vilib>:"Conv_Meters_Feet.vi"("Meters"=w734) -> ("Feet"=w733:dbl)  [unwired: 10 in]
                n298 = call <vilib>:"Conv_Meters_Feet.vi"("Meters"=w736) -> ("Feet"=w735:dbl)  [unwired: 10 in]
                n299 = call <vilib>:"Conv_Meters_Feet.vi"("Meters"=w737) -> ("Feet"=w730:dbl)  [unwired: 10 in]
                n300 = call <vilib>:"Conv_Meters_Feet.vi"("Meters"=1.0 ("Centimeter")) -> ("Feet"=w727:dbl)  [unwired: 10 in]
                n301 = Divide(x=w726, y=w727) -> (x/y=w725:dbl)
                n302 = in-place-cluster #15("Acceleration"=w731, "TimeSeconds"=w740, "Velocity"=w733, "Curvature"=w725, "POSE.TRANSLATION.X"=w735, "POSE.TRANSLATION.Y"=w730, "POSE.ROTATION.VALUE"=w729, "POSE.ROTATION.COS"=w739, "POSE.ROTATION.SIN"=w738) -> (w723:T7)
              }
            }
          }
          frame "Radio Selection 5" {
            # "Meters - Conv to Inches"
            n303 = for {
              tunnel: w742 -> [w744] mode=indexing
              tunnel: [w743] -> w741 mode=indexing
              n304 = in-place {
                n305 = in-place-cluster #16(w744) -> ("Acceleration"=w752:dbl, "TimeSeconds"=w760:dbl, "Velocity"=w754:dbl, "Curvature"=w746:dbl, "POSE.TRANSLATION.X"=w756:dbl, "POSE.TRANSLATION.Y"=w757:dbl, "POSE.ROTATION.VALUE"=w749:dbl, "POSE.ROTATION.COS"=w759:dbl, "POSE.ROTATION.SIN"=w758:dbl)
                n306 = call <vilib>:"Conv_Meters_Inches.vi"("Meters"=w752) -> ("Inches"=w751:dbl)  [unwired: 10 in]
                n307 = call <vilib>:"Conv_Meters_Inches.vi"("Meters"=w754) -> ("Inches"=w753:dbl)  [unwired: 10 in]
                n308 = call <vilib>:"Conv_Meters_Inches.vi"("Meters"=w756) -> ("Inches"=w755:dbl)  [unwired: 10 in]
                n309 = call <vilib>:"Conv_Meters_Inches.vi"("Meters"=w757) -> ("Inches"=w750:dbl)  [unwired: 10 in]
                n310 = call <vilib>:"Conv_Meters_Inches.vi"("Meters"=1.0 ("Centimeter")) -> ("Inches"=w747:dbl)  [unwired: 10 in]
                n311 = Divide(x=w746, y=w747) -> (x/y=w745:dbl)
                n312 = in-place-cluster #16("Acceleration"=w751, "TimeSeconds"=w760, "Velocity"=w753, "Curvature"=w745, "POSE.TRANSLATION.X"=w755, "POSE.TRANSLATION.Y"=w750, "POSE.ROTATION.VALUE"=w749, "POSE.ROTATION.COS"=w759, "POSE.ROTATION.SIN"=w758) -> (w743:T7)
              }
            }
          }
        }
        n313 = call <vilib>:"Trajectory_New.vi"("TRAJ_STATES"=w630) -> ("TRAJECTORY"=w631:T13)  [unwired: 10 in]
        n314 = Path To String(path="Trajectory JSON File Name") -> (string=w636:string)
        n315 = call <vilib>:"TrajectoryUtil_toPathWeaverJSON.vi"("inTRAJECTORY"=w631, "FileName"=w636) -> ("error out"=w637:errorcluster)  [unwired: 9 in]
        "Write CSV File Error" <- w637
        n316 = case shown="Error .." w637 {
          tunnel: [TRUE ("File Saved\nWithout\nError") FALSE ("File Saved\nWithout\nError")] -> w640
          frame No Error {
          }
          frame Error {
          }
        }
      }
      frame 5 {
        # "write xml\nfile"
        # "convert\nto xml\nstring"
        # "Write config to File"
        n317 = Bundle By Name(cluster=T14 {"Write Config File Name"=path "", "Write Config File Comment"="", "WayPoints"=[], "TRAJECTORY_CONFIG"={"MaxVelocity"=0.0, "Max Acceleration"=0.0, "StartVelocity"=0.0, "End Velocity"=0.0, "Reversed"=FALSE, "DiffDrKineConstntDefined"=FALSE, "CentAcellConstntDefined"=FALSE, "DiffDrVoltConstntDefined"=FALSE, "DIFF_DRIVE_KINE_CONSTRAINT"={"Max Speed (M/S)"=0.0, "DIFF_DRIVE_KINEMATICS"={"TrackWidth_Meters"=0.0}}, "CENTRIPETAL_ACCEL_CONSTRAINT"={"Max Cent Accel"=0.0}, "SwerveDrKineConstntDefined"=FALSE, "SWERVE_DRIVE_KINE_CONSTRAINT"={"Max Speed (M/S)"=0.0, "SwerveKinematics"={"NumModules"=0, "InverseKinematics"=[], "ForwardKinematics"=[], "Modules"=[], "PrevCoR"={"X"=0.0, "Y"=0.0}}}, "DIFF_DRIVE_VOLTAGE_CONSTRAINT"={"Max Voltage"=0.0, "DIFF_DRIVE_KINEMATICS"={"TrackWidth_Meters"=0.0}, "SIMPLE_MOTOR_FF"={"Ks"=0.0, "Kv"=0.0, "Ka"=0.0}}, "MECANUM_DRIVE_KINE_CONSTRAINT"={"Max Speed (M/S)"=0.0, "MECA_DRIVE_KINEMATICS"={"FrontLeft"={"X"=0.0, "Y"=0.0}, "FrontRight"={"X"=0.0, "Y"=0.0}, "RearLeft"={"X"=0.0, "Y"=0.0}, "RearRight"={"X"=0.0, "Y"=0.0}, "InverseKinematics"=[], "ForwardKinematics"=[], "PrevCoR"={"X"=0.0, "Y"=0.0}}}, "MecanumDrKineConstntDefined"=FALSE}, "IsCubic"=FALSE, "Units Selector"=enum."Inches", "UseWeights"=FALSE} ("TrajCreateConfig"), "Write Config File Name"="Write Config File Name", "Write Config File Comment"="Write Config File Comment", "WayPoints"=w782, "TRAJECTORY_CONFIG"=w781, "IsCubic"=w780, "Units Selector"=w771, "UseWeights"=w769) -> (w778:T14)
        n318 = local write "Trajectory File Comment"("Write Config File Comment") -> ()
        n319 = Flatten To XML(anything=w778) -> (xml string=w776:string)
        n320 = call-poly <vilib>:"Write to XML File.vi"("Standalone? (T)"=TRUE, "XML Input"=w776, "XML File Path"="Write Config File Name") -> ("error out"=w774:errorcluster)  [unwired: 6 in, 2 out]
        "Write Config FIle Error" <- w774
        n321 = case shown="No Error" w774 {
          tunnel: [TRUE ("File Saved\nWithout\nError") FALSE ("File Saved\nWithout\nError")] -> w773
          frame No Error {
          }
          frame Error {
          }
        }
      }
      frame 6 {
        # "End Program"
        n322 = disable-structure shown="Default" {
          frame condition #0 (active) {
            n323 = Stop() -> ()  [unwired: 1 in]
          }
          frame condition #1 {
            n324 = Quit LabVIEW() -> ()  [unwired: 1 in]
          }
        }
      }
    }
    "Trajectory\nCompleted\nError Free" <- w78
    "CSV File Saved\nWithout Error" <- w74
    "Config File Saved\nWithout Error" <- w27
    "JSON File Saved\nWithout Error" <- w12
  }
